vi "plcHMI_rev5.vi"() -> ()   [LabVIEW 2020]
doc: "ADS continuos synchronous write example using base blocks. \n\nThe client writes data synchronously and does wait for the respose from server."
uses:
  Agilent/AgilentTotalCluster.ctl
  Agilent/AgilentControl.ctl
  Agilent/Channel Config.ctl
  <vilib>/Platform/TimedLoop/XDataNode/timing_clust.ctl
  <vilib>/Platform/TimedLoop/XDataNode/nitl_modes.ctl
  <vilib>/Platform/TimedLoop/XDataNode/wakeup.ctl
  <userlib>/Beckhoff-LabVIEW-Interface/_DependsOn/With TypeResolving/Write Sync Single TypeResolved.vi
  <userlib>/Beckhoff-LabVIEW-Interface/_DependsOn/With TypeResolving/Read Sync Single TypeResolved.vi
  <vilib>/Platform/TimedLoop/XDataNode/XDataNode.xnode
  <vilib>/Platform/TimedLoop/XDataNode/XDNodeRunTimeDep.lvlib
panel:
  in  "Tab Control":T1(tab)
  out "error out":errorcluster
  in  "Symbol file path - MUST BE ENTERED\nLoad \"ADS Write AND Read Symbols REV X.X.xml\"":path
  out "bHasMached":bool
  out "Write Status":bool
  out "Read Status":bool
  in  "EXIT HMI":bool caption="STOP HMI\nEXIT HMI"
  out "Internal TwinCAT Handle ID Maps":dbl format="%#_12g"
  in  "802L TDK PSU Voltage Rating (abs(Volts))":i32=12000 min=1 max=50000
  in  "802L TDL PSU Peak Power (J/s)":i32=9000 min=1 max=50000
  in  "HVPS Model":u16(ring) items=["802L-12kV,9000J/s", "802L+50kV,9000J/s", "Other"]
  out "Test Interval Fault":bool
  in  "Cycle Time (Sec)":i32=15 min=0
  in  "Voltage Held by PSU":bool
  in  "Log Capacitor Voltage":bool
  in  "Log Temperature Data":bool
  out "Time Since Last Shot":string caption="Elapsed Time Text"
  in  "Duty Cycle":dbl
  in  "Current Control":bool
  out "Expected Voltage":i16
  in  "Dump":bool
  out "EOC":bool
  out "Maximum Test Number Reached":bool
  out "SCR Ready":bool
  in  "START":bool
  in  "STOP":bool
  in  "Hold":bool
  in  "Charge":bool
  in  "Shot":bool
  in  "HV Switch Mode":bool
  in  "CLEAR FAULT":bool
  in  "Manual/Auto":bool=TRUE
  out "Test Interval (Sec)":i32=15 min=0
  in  "Capacitance (uF)":sgl=1e-13 min=0 max=10000 format="%#_6f"
  in  "Target Charge Volt (V) - Min 1500V - TEMPORARY LIMIT 12kV":i32 min=-12000 max=12000 step=1
  out "Estimated Charge Time (seconds)":sgl
  in  "Hold Time Before Shot (seconds)":sgl max=1000
  in  "Max Number of Shots (Test intervals)":i16=1 min=1
  out "Shot Number":i16
  out "Charge Fault":bool=TRUE
  out "Discharge Fault":bool=TRUE
  out "Hold Fault":bool=TRUE
  out "Cap 1 Temp\nExceeded Fault":bool=TRUE
  out "Ambient Temp\nExceeded Fault":bool=TRUE
  out "PSU Fault":bool=TRUE
  out "Control Sys Fault":bool=TRUE
  out "test Running":bool
  out "Test State":string
  out "Cap 1 Voltage":i16
  out "Cap 1 Temperature":i16
  in  "Capacitor Voltage Data Log File Path (.xlsx)":path
  out "Load Temperature":i16
  out "Soft Dump Temp":i16
  out "Ambient Temp":i16
  out "Waveform Chart - Capacitor Voltage (Probe, abs(Volts))":dbl(graph)
  in  "Manual Charge Time (seconds)":sgl max=90
  in  "Reset Test Number":bool
  in  "Cap 1 Fault Temp (Cel)":i16 min=0 max=125
  in  "Capacitor Temperature Data Log File Path (.xlsx)":path
  out "Cap 1 Voltage (HVPS)":i16
  out "Capacitor Voltage":cluster{dbl, dbl}(graph)
  out "EOC":i16(graph)
  out "Soft Exception":bool
  out "PSU HV FB Fault":bool
  out "Charge FB Fault":bool
  out "Softdump FB Fault":bool
  out "SCR FB":i16(graph)
  out "Spark Gap Voltage":i16(graph)
  in  "CH4 Vertical Units":string(combo)="V"
  in  "CH4 Vertical Units/div":dbl=2.0
  in  "Toggle Scope Scale":bool
  in  "CH1 Vertical Units/div":dbl=2.0
  in  "CH1 Vertical Units":string(combo)="V"
  in  "Horizontal Units":enum16{"us", "ms", "s"}(ring)
  in  "Horizontal Units/div":dbl=200.0
  out "Download":bool
  in  "Single":bool
  in  "Stop":bool
  out "Scope Trig":bool
  in  "Agilent Array":T2[](array[typedef])
  out "Process Step":u8
  out "Stop Loops":bool
  # "CONFIGURATION"
  # "Press STOP HMI instead of\nLabView Abort Execution"
  # "PSU V Rating, Peak Power\nactive when OTHER\nis selected"
  # "INPUT VARIABLES - For TDK Lambda 802L\nMust be written to before START"
  # "FAULT STATUSES"
  # "Set to -1 for automated\nfull charge to setpoint"
  # "MANUAL CONTROLS"
  # "Does not record during \"wait\" and appends to data file. Must be named with .xlsx"
  # "HV Switch Configuration"
  # "Records during \"Test Running.\" Must be named with .xlsx"
  # "Control Sys Faults"
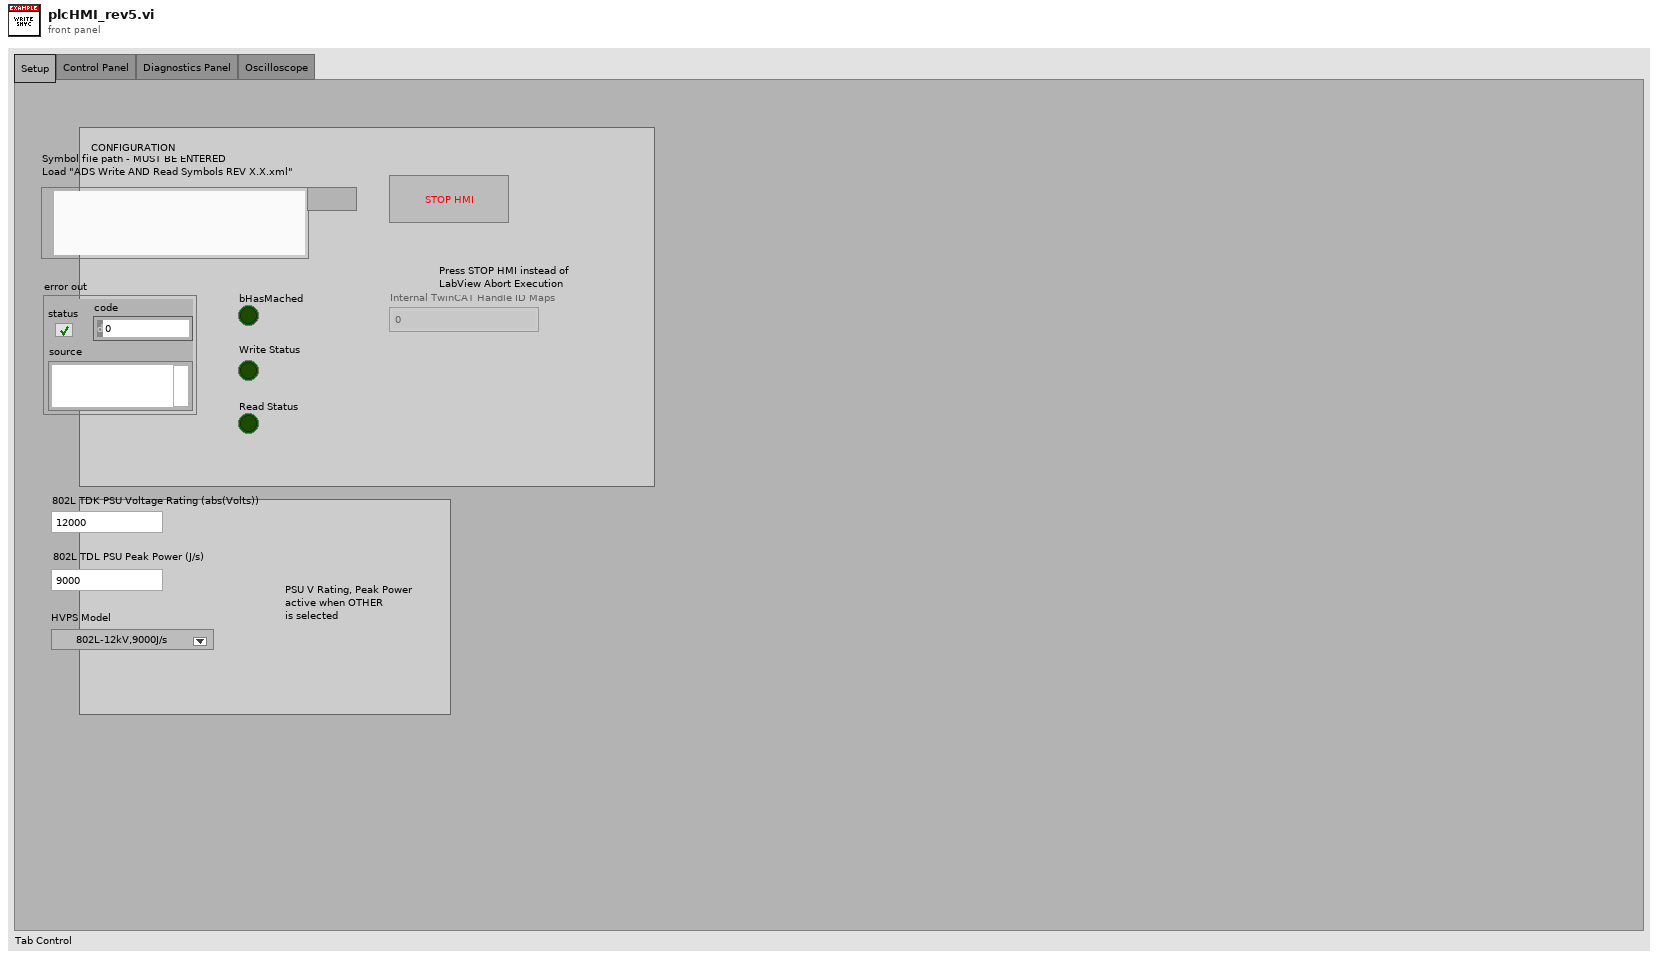
[diagram p1: front panel]
types:
  T1 = enum32{"Setup", "Control Panel", "Diagnostics Panel", "Oscilloscope"}
  T2 = typedef "AgilentTotalCluster.ctl" = cluster{"Agilent Graph":waveform(dbl)[], "Agilent Control":T3, "Agilent Setup Error":errorcluster, "Agilent Present":bool, "Enabled":bool}
  T3 = typedef "AgilentControl.ctl" = cluster{"Trig?":bool, "VISA session":refnum<visa-resource-name>, "Setup to Load":string, "Timeout (ms)":u32, "Desired Samp":enum32{"100", "250", "500", "1000", "2000", "5000", "10000", "20000", "50000", "100000", "200000", "500000", "1000000", "2000000", "4000000", "8000000"}, "Captured Samp":i32, "Desired Channels":T4[]}
  T4 = typedef "Channel Config.ctl" = cluster{"Chan Index":enum16{"Channel1", "Channel2", "Channel3", "Channel4", "MATH"}, "Name":string, "Samples":i32}
  T5 = typedef "XDNodeRunTimeDep.lvlib/timing_clust.ctl" = cluster{"Expected End [f-1]":u64, "Actual End [f-1]":u64, "Finished Late? [f-1]":bool, "Expected End [i-1]":u64, "Actual End [i-1]":u64, "Finished Late? [i-1]":bool, "Expected Start [i]":u64, "Actual Start [i]":u64, "Expected Start [f]":u64, "Actual Start [f]":u64, "Source Name":string, "Structure Name":string, "Period":i64, "Deadline":i64, "Offset":i64, "Start":i64, "Priority":i32, "Timeout":i32, "Mode":T6, "Wakeup Reason":T7, "Error":errorcluster, "Source Type":string, "Secondary Source Type":string, "Global End Time":u64, "Global Start Time":u64, "Frame Duration":u64, "Iteration Duration":u64, "Assigned CPU":i32, "I/O Scan Engine Mode":u32}
  T6 = typedef "XDNodeRunTimeDep.lvlib/nitl_modes.ctl" = enum32{"No Change", "Process missed periods, maintain original phase", "Discard missed periods, maintain original phase", "Process missed periods, ignore original phase", "Discard missed periods, ignore original phase"}
  T7 = typedef "XDNodeRunTimeDep.lvlib/wakeup.ctl" = enum32{"Normal", "Aborted", "Asynchronous wakeup", "Timing source error", "Timed loop error", "Timeout"}
  T8 = cluster{"Agilent Array[0]":T2, "Agilent Array[1]":T2, "Agilent Array[2]":T2, "Agilent Array[3]":T2, "Agilent Array[4]":T2, "Agilent Array[5]":T2, "Agilent Array[6]":T2, "Agilent Array[7]":T2, "Agilent Array[8]":T2}
  T9 = enum32{"100", "250", "500", "1000", "2000", "5000", "10000", "20000", "50000", "100000", "200000", "500000", "1000000", "2000000", "4000000", "8000000"}
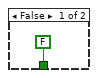
[diagram p2: hidden frame]
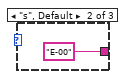
[diagram p5: hidden frame]
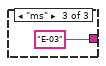
[diagram p6: hidden frame]
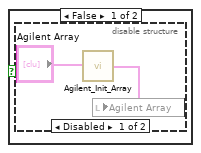
[diagram p7: hidden frame]
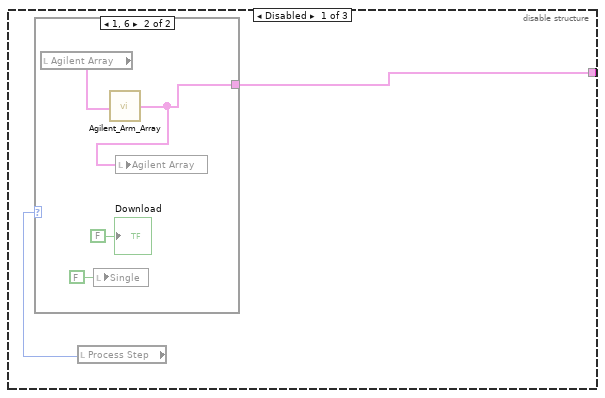
[diagram p11: hidden frame]
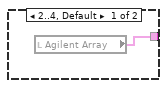
[diagram p12: hidden frame]
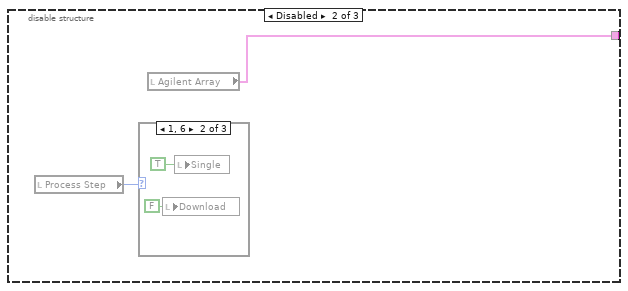
[diagram p13: hidden frame]
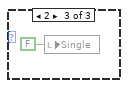
[diagram p15: hidden frame]
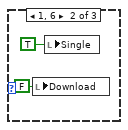
[diagram p17: hidden frame]
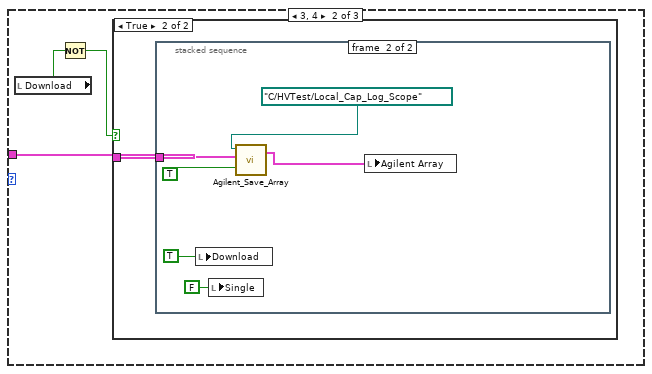
[diagram p19: hidden frame]
diagram:
  w91 = u16 17 items=["SyncLatest"=17, "AsyncLatest"=33] ("WriterMode")
  w161 = u16 33 items=["SyncLatest"=17, "AsyncLatest"=33] ("WriterMode")
  w201 = u16 33 items=["SyncLatest"=17, "AsyncLatest"=33] ("WriterMode")
  w220 = u16 33 items=["SyncLatest"=17, "AsyncLatest"=33] ("WriterMode")
  w239 = u16 33 items=["SyncLatest"=17, "AsyncLatest"=33] ("WriterMode")
  w258 = u16 33 items=["SyncLatest"=17, "AsyncLatest"=33] ("WriterMode")
  w277 = u16 33 items=["SyncLatest"=17, "AsyncLatest"=33] ("WriterMode")
  w296 = u16 17 items=["SyncLatest"=17, "AsyncLatest"=33] ("WriterMode")
  w315 = u16 17 items=["SyncLatest"=17, "AsyncLatest"=33] ("WriterMode")
  w334 = u16 17 items=["SyncLatest"=17, "AsyncLatest"=33] ("WriterMode")
  w353 = u16 17 items=["SyncLatest"=17, "AsyncLatest"=33] ("WriterMode")
  w372 = u16 17 items=["SyncLatest"=17, "AsyncLatest"=33] ("WriterMode")
  w391 = u16 17 items=["SyncLatest"=17, "AsyncLatest"=33] ("WriterMode")
  w410 = u16 17 items=["SyncLatest"=17, "AsyncLatest"=33] ("WriterMode")
  w425 = u16 17 items=["SyncLatest"=17, "AsyncLatest"=33] ("WriterMode")
  # "Variables/ Control"
  # "Documentation:\nCode separated vertically into two main sections - Write and read\nThey are further separated into BOOL and numeric\nThe OR gates wire all the error lines and the EXIT HMI button to a WHILE LOOP STOP\nThere current delay time on the routine is 100ms\nAll the AND gates connect the typecast resolve lines to the bHasMatched indicator\nThe second and third set of AND gates connect the write statuses to the Write Status indicator\nThe same is done for the read status indicator"
  # "WRITE NUMERICS"
  # "WRITE BOOLS"
  # "Select Symbol N"
  # "Read Initialization"
  # "Release \nTypeResolver"
  # "Release Writer"
  # "Send Request"
  # "Init \nTypeResolver"
  # "Init Writer"
  # "Select Symbol"
  # "Initialization"
  # "Call Release handle block\nat the end, when all nodes\nhave finished their execution"
  # "There must be only one release\nafter every init block.\nRelease block must be called\nalways at the end."
  # "Release"
  # "Symbol Interface"
  n1 = disable-structure shown="Enabled" {
    disable-tunnel: [w431 _] -> w429
    disable-tunnel: [w430 w433] -> w428
    frame Disabled {
      # "Using Symbol Interface"
      n2 = call <userlib>:"Symbol Interface.vi"() -> ("PortInfo"=w430:string, "error out"=w431:errorcluster)  [unwired: 14 in]
    }
    frame Enabled {
      # "Using Symbol File"
      n3 = Path To String(path="Symbol file path - MUST BE ENTERED\nLoad \"ADS Write AND Read Symbols REV X.X.xml\"") -> (string=w433:string)
    }
  }
  n4 = call <userlib>:"Init.vi"("XMLDescription"=w428, "error in (no error)"=w429) -> ("Handle"=w41:u32, "ReadGrpSymbols"=w5:string[], "WriteGrpSymbols"=w29:string[], "error out"=w7:errorcluster)  [unwired: 9 in, 1 out]
  n5 = Index Array(array=w29, index=0) -> (element=w18:string)
  n6 = Index Array(array=w29, index=21) -> (element=w28:string)
  n7 = Index Array(array=w29, index=20) -> (element=w34:string)
  n8 = Index Array(array=w29, index=14) -> (element=w8:string)
  n9 = Index Array(array=w29, index=9) -> (element=w278:string)
  n10 = Index Array(array=w29, index=10) -> (element=w259:string)
  n11 = Index Array(array=w29, index=12) -> (element=w221:string)
  n12 = Index Array(array=w29, index=11) -> (element=w240:string)
  n13 = Index Array(array=w29, index=13) -> (element=w202:string)
  n14 = Index Array(array=w29, index=18) -> (element=w42:string)
  n15 = Index Array(array=w29, index=19) -> (element=w35:string)
  n16 = Index Array(array=w29, index=7) -> (element=w297:string)
  n17 = Index Array(array=w29, index=2) -> (element=w392:string)
  n18 = Index Array(array=w29, index=3) -> (element=w373:string)
  n19 = Index Array(array=w29, index=5) -> (element=w335:string)
  n20 = Index Array(array=w29, index=4) -> (element=w354:string)
  n21 = Index Array(array=w29, index=6) -> (element=w316:string)
  n22 = Index Array(array=w29, index=1) -> (element=w411:string)
  n23 = Index Array(array=w29, index=16) -> (element=w11:string)
  n24 = Index Array(array=w29, index=8) -> (element=w90:string)
  n25 = Index Array(array=w29, index=15) -> (element=w162:string)
  n26 = Index Array(array=w29, index=17) -> (element=w13:string)
  n27 = call <userlib>:"Init Writer.vi"("Handle"=w41, "SymbolName"=w278, "WriterMode"=w277, "error constant"=w7) -> ("Handle"=w273:u32, "SymbolName"=w272:string, "WriterMode"=w271:u16, "WriteHandle"=w269:u32, "error IO"=w270:errorcluster)  [unwired: 7 in]
  n28 = call <userlib>:"Init Writer.vi"("Handle"=w41, "SymbolName"=w259, "WriterMode"=w258, "error constant"=w7) -> ("Handle"=w257:u32, "SymbolName"=w256:string, "WriterMode"=w255:u16, "WriteHandle"=w254:u32, "error IO"=w253:errorcluster)  [unwired: 7 in]
  n29 = call <userlib>:"Init Writer.vi"("Handle"=w41, "SymbolName"=w221, "WriterMode"=w220, "error constant"=w7) -> ("Handle"=w219:u32, "SymbolName"=w218:string, "WriterMode"=w217:u16, "WriteHandle"=w216:u32, "error IO"=w215:errorcluster)  [unwired: 7 in]
  n30 = call <userlib>:"Init Type.vi"("Handle"=w41, "SymbolName"=w278, "error in"=w7) -> ("Handle"=w262:u32, "TypeHdl"=w261:u32, "error IO"=w260:errorcluster)  [unwired: 7 in, 3 out]
  n31 = call <userlib>:"Init Type.vi"("Handle"=w41, "SymbolName"=w259, "error in"=w7) -> ("Handle"=w252:u32, "TypeHdl"=w251:u32, "error IO"=w250:errorcluster)  [unwired: 7 in, 3 out]
  n32 = call <userlib>:"Init Writer.vi"("Handle"=w41, "SymbolName"=w240, "WriterMode"=w239, "error constant"=w7) -> ("Handle"=w238:u32, "SymbolName"=w237:string, "WriterMode"=w236:u16, "WriteHandle"=w235:u32, "error IO"=w234:errorcluster)  [unwired: 7 in]
  n33 = call <userlib>:"Init Type.vi"("Handle"=w41, "SymbolName"=w221, "error in"=w7) -> ("Handle"=w214:u32, "TypeHdl"=w213:u32, "error IO"=w212:errorcluster)  [unwired: 7 in, 3 out]
  n34 = call <userlib>:"Init Writer.vi"("Handle"=w41, "SymbolName"=w202, "WriterMode"=w201, "error constant"=w7) -> ("Handle"=w200:u32, "SymbolName"=w199:string, "WriterMode"=w198:u16, "WriteHandle"=w197:u32, "error IO"=w196:errorcluster)  [unwired: 7 in]
  n35 = call <userlib>:"Init Type.vi"("Handle"=w41, "SymbolName"=w240, "error in"=w7) -> ("Handle"=w233:u32, "TypeHdl"=w232:u32, "error IO"=w231:errorcluster)  [unwired: 7 in, 3 out]
  n36 = call <userlib>:"Init Type.vi"("Handle"=w41, "SymbolName"=w202, "error in"=w7) -> ("Handle"=w195:u32, "TypeHdl"=w194:u32, "error IO"=w193:errorcluster)  [unwired: 7 in, 3 out]
  n37 = call <userlib>:"Init Writer.vi"("Handle"=w41, "SymbolName"=w297, "WriterMode"=w296, "error constant"=w7) -> ("Handle"=w295:u32, "SymbolName"=w294:string, "WriterMode"=w293:u16, "WriteHandle"=w292:u32, "error IO"=w291:errorcluster)  [unwired: 7 in]
  n38 = call <userlib>:"Init Writer.vi"("Handle"=w41, "SymbolName"=w392, "WriterMode"=w391, "error constant"=w7) -> ("Handle"=w387:u32, "SymbolName"=w386:string, "WriterMode"=w385:u16, "WriteHandle"=w383:u32, "error IO"=w384:errorcluster)  [unwired: 7 in]
  n39 = call <userlib>:"Init Writer.vi"("Handle"=w41, "SymbolName"=w373, "WriterMode"=w372, "error constant"=w7) -> ("Handle"=w371:u32, "SymbolName"=w370:string, "WriterMode"=w369:u16, "WriteHandle"=w368:u32, "error IO"=w367:errorcluster)  [unwired: 7 in]
  n40 = call <userlib>:"Init Writer.vi"("Handle"=w41, "SymbolName"=w335, "WriterMode"=w334, "error constant"=w7) -> ("Handle"=w333:u32, "SymbolName"=w332:string, "WriterMode"=w331:u16, "WriteHandle"=w330:u32, "error IO"=w329:errorcluster)  [unwired: 7 in]
  n41 = call <userlib>:"Init Type.vi"("Handle"=w41, "SymbolName"=w297, "error in"=w7) -> ("Handle"=w290:u32, "TypeHdl"=w289:u32, "error IO"=w288:errorcluster)  [unwired: 7 in, 3 out]
  n42 = call <userlib>:"Init Type.vi"("Handle"=w41, "SymbolName"=w392, "error in"=w7) -> ("Handle"=w376:u32, "TypeHdl"=w375:u32, "error IO"=w374:errorcluster)  [unwired: 7 in, 3 out]
  n43 = call <userlib>:"Init Type.vi"("Handle"=w41, "SymbolName"=w373, "error in"=w7) -> ("Handle"=w366:u32, "TypeHdl"=w365:u32, "error IO"=w364:errorcluster)  [unwired: 7 in, 3 out]
  n44 = call <userlib>:"Init Writer.vi"("Handle"=w41, "SymbolName"=w354, "WriterMode"=w353, "error constant"=w7) -> ("Handle"=w352:u32, "SymbolName"=w351:string, "WriterMode"=w350:u16, "WriteHandle"=w349:u32, "error IO"=w348:errorcluster)  [unwired: 7 in]
  n45 = call <userlib>:"Init Type.vi"("Handle"=w41, "SymbolName"=w335, "error in"=w7) -> ("Handle"=w328:u32, "TypeHdl"=w327:u32, "error IO"=w326:errorcluster)  [unwired: 7 in, 3 out]
  n46 = call <userlib>:"Init Writer.vi"("Handle"=w41, "SymbolName"=w316, "WriterMode"=w315, "error constant"=w7) -> ("Handle"=w314:u32, "SymbolName"=w313:string, "WriterMode"=w312:u16, "WriteHandle"=w311:u32, "error IO"=w310:errorcluster)  [unwired: 7 in]
  n47 = call <userlib>:"Init Type.vi"("Handle"=w41, "SymbolName"=w354, "error in"=w7) -> ("Handle"=w347:u32, "TypeHdl"=w346:u32, "error IO"=w345:errorcluster)  [unwired: 7 in, 3 out]
  n48 = call <userlib>:"Init Type.vi"("Handle"=w41, "SymbolName"=w316, "error in"=w7) -> ("Handle"=w309:u32, "TypeHdl"=w308:u32, "error IO"=w307:errorcluster)  [unwired: 7 in, 3 out]
  n49 = call <userlib>:"Init Writer.vi"("Handle"=w41, "SymbolName"=w411, "WriterMode"=w410, "error constant"=w7) -> ("Handle"=w409:u32, "SymbolName"=w408:string, "WriterMode"=w407:u16, "WriteHandle"=w406:u32, "error IO"=w405:errorcluster)  [unwired: 7 in]
  n50 = call <userlib>:"Init Type.vi"("Handle"=w41, "SymbolName"=w411, "error in"=w7) -> ("Handle"=w404:u32, "TypeHdl"=w403:u32, "error IO"=w402:errorcluster)  [unwired: 7 in, 3 out]
  n51 = call <userlib>:"Init Writer.vi"("Handle"=w41, "SymbolName"=w18, "WriterMode"=w425, "error constant"=w7) -> ("Handle"=w424:u32, "SymbolName"=w423:string, "WriterMode"=w422:u16, "WriteHandle"=w421:u32, "error IO"=w420:errorcluster)  [unwired: 7 in]
  n52 = call <userlib>:"Init Type.vi"("Handle"=w41, "SymbolName"=w18, "error in"=w7) -> ("Handle"=w419:u32, "TypeHdl"=w418:u32, "error IO"=w413:errorcluster)  [unwired: 7 in, 3 out]
  n53 = call <userlib>:"Init Writer.vi"("Handle"=w41, "SymbolName"=w162, "WriterMode"=w161, "error constant"=w7) -> ("Handle"=w157:u32, "SymbolName"=w156:string, "WriterMode"=w155:u16, "WriteHandle"=w147:u32, "error IO"=w154:errorcluster)  [unwired: 7 in]
  n54 = call <userlib>:"Init Type.vi"("Handle"=w41, "SymbolName"=w162, "error in"=w7) -> ("Handle"=w152:u32, "TypeHdl"=w150:u32, "error IO"=w151:errorcluster)  [unwired: 7 in, 3 out]
  n55 = Index Array(array=w5, index=2) -> (element=w143:string)
  n56 = Index Array(array=w5, index=4) -> (element=w139:string)
  n57 = call <userlib>:"Init Writer.vi"("Handle"=w41, "SymbolName"=w90, "WriterMode"=w91, "error constant"=w7) -> ("Handle"=w89:u32, "SymbolName"=w88:string, "WriterMode"=w87:u16, "WriteHandle"=w86:u32, "error IO"=w85:errorcluster)  [unwired: 7 in]
  n58 = Index Array(array=w5, index=1) -> (element=w179:string)
  n59 = Index Array(array=w5, index=21) -> (element=w56:string)
  n60 = Index Array(array=w5, index=22) -> (element=w53:string)
  n61 = call <userlib>:"Init Type.vi"("Handle"=w41, "SymbolName"=w90, "error in"=w7) -> ("Handle"=w84:u32, "TypeHdl"=w83:u32, "error IO"=w82:errorcluster)  [unwired: 7 in, 3 out]
  n62 = Index Array(array=w5, index=0) -> (element=w178:string)
  n63 = Index Array(array=w5, index=3) -> (element=w140:string)
  n64 = Index Array(array=w5, index=20) -> (element=w61:string)
  n65 = Index Array(array=w5, index=23) -> (element=w52:string)
  n66 = Index Array(array=w5, index=16) -> (element=w145:string)
  n67 = Index Array(array=w5, index=24) -> (element=w50:string)
  n68 = Index Array(array=w5, index=28) -> (element=w3:string)
  n69 = Index Array(array=w5, index=11) -> (element=w167:string)
  n70 = Index Array(array=w5, index=10) -> (element=w168:string)
  n71 = Index Array(array=w5, index=17) -> (element=w64:string)
  n72 = Index Array(array=w5, index=18) -> (element=w63:string)
  n73 = Index Array(array=w5, index=13) -> (element=w165:string)
  n74 = Index Array(array=w5, index=27) -> (element=w22:string)
  n75 = Index Array(array=w5, index=12) -> (element=w166:string)
  n76 = Index Array(array=w5, index=15) -> (element=w163:string)
  n77 = Index Array(array=w5, index=19) -> (element=w62:string)
  n78 = Index Array(array=w5, index=26) -> (element=w23:string)
  n79 = Index Array(array=w5, index=5) -> (element=w75:string)
  n80 = Index Array(array=w5, index=6) -> (element=w133:string)
  n81 = Index Array(array=w5, index=9) -> (element=w177:string)
  n82 = Index Array(array=w5, index=14) -> (element=w164:string)
  n83 = Index Array(array=w5, index=8) -> (element=w135:string)
  n84 = Index Array(array=w5, index=25) -> (element=w39:string)
  n85 = Index Array(array=w5, index=7) -> (element=w134:string)
  n86 = node-c288(i64 10 ("Period")) -> (w99:T5)  [unwired: 2 in]
  n87 = timed-loop {
    tunnel: w424 -> [w741]
    tunnel: w423 -> [w740]
    tunnel: w422 -> [w739]
    tunnel: w421 -> [w738]
    tunnel: w419 -> [w983]
    tunnel: w418 -> [w982]
    tunnel: [w736] -> w417
    tunnel: [w735] -> w416
    tunnel: [w981] -> w415
    tunnel: [w980] -> w414
    tunnel: w409 -> [w978]
    tunnel: w408 -> [w977]
    tunnel: w407 -> [w976]
    tunnel: w406 -> [w975]
    tunnel: w404 -> [w973]
    tunnel: w403 -> [w972]
    tunnel: [w970] -> w400
    tunnel: [w969] -> w399
    tunnel: [w968] -> w397
    tunnel: [w967] -> w396
    tunnel: w387 -> [w966]
    tunnel: w386 -> [w965]
    tunnel: w385 -> [w964]
    tunnel: w383 -> [w962]
    tunnel: [w961] -> w382
    tunnel: [w960] -> w381
    tunnel: [w959] -> w378
    tunnel: [w958] -> w377
    tunnel: w376 -> [w957]
    tunnel: w375 -> [w956]
    tunnel: w371 -> [w954]
    tunnel: w370 -> [w953]
    tunnel: w369 -> [w952]
    tunnel: w368 -> [w951]
    tunnel: w366 -> [w949]
    tunnel: w365 -> [w948]
    tunnel: [w946] -> w362
    tunnel: [w945] -> w361
    tunnel: [w944] -> w359
    tunnel: [w943] -> w358
    tunnel: w352 -> [w942]
    tunnel: w351 -> [w941]
    tunnel: w350 -> [w940]
    tunnel: w349 -> [w939]
    tunnel: w347 -> [w937]
    tunnel: w346 -> [w936]
    tunnel: [w934] -> w343
    tunnel: [w933] -> w342
    tunnel: [w932] -> w340
    tunnel: [w931] -> w339
    tunnel: w333 -> [w930]
    tunnel: w332 -> [w929]
    tunnel: w331 -> [w928]
    tunnel: w330 -> [w927]
    tunnel: w328 -> [w925]
    tunnel: w327 -> [w924]
    tunnel: [w922] -> w324
    tunnel: [w921] -> w323
    tunnel: [w920] -> w321
    tunnel: [w919] -> w320
    tunnel: w314 -> [w918]
    tunnel: w313 -> [w917]
    tunnel: w312 -> [w916]
    tunnel: w311 -> [w915]
    tunnel: w309 -> [w913]
    tunnel: w308 -> [w912]
    tunnel: [w910] -> w305
    tunnel: [w909] -> w304
    tunnel: [w908] -> w302
    tunnel: [w907] -> w301
    tunnel: w295 -> [w906]
    tunnel: w294 -> [w905]
    tunnel: w293 -> [w904]
    tunnel: w292 -> [w903]
    tunnel: w290 -> [w901]
    tunnel: w289 -> [w900]
    tunnel: [w898] -> w286
    tunnel: [w897] -> w285
    tunnel: [w896] -> w283
    tunnel: [w895] -> w282
    tunnel: w273 -> [w894]
    tunnel: w272 -> [w893]
    tunnel: w271 -> [w892]
    tunnel: w269 -> [w890]
    tunnel: [w889] -> w268
    tunnel: [w888] -> w267
    tunnel: [w887] -> w264
    tunnel: [w886] -> w263
    tunnel: w262 -> [w885]
    tunnel: w261 -> [w884]
    tunnel: w257 -> [w882]
    tunnel: w256 -> [w881]
    tunnel: w255 -> [w880]
    tunnel: w254 -> [w879]
    tunnel: w252 -> [w877]
    tunnel: w251 -> [w876]
    tunnel: [w874] -> w248
    tunnel: [w873] -> w247
    tunnel: [w872] -> w245
    tunnel: [w871] -> w244
    tunnel: w238 -> [w870]
    tunnel: w237 -> [w869]
    tunnel: w236 -> [w868]
    tunnel: w235 -> [w867]
    tunnel: w233 -> [w865]
    tunnel: w232 -> [w864]
    tunnel: [w862] -> w229
    tunnel: [w861] -> w228
    tunnel: [w860] -> w226
    tunnel: [w859] -> w225
    tunnel: w219 -> [w858]
    tunnel: w218 -> [w857]
    tunnel: w217 -> [w856]
    tunnel: w216 -> [w855]
    tunnel: w214 -> [w853]
    tunnel: w213 -> [w852]
    tunnel: [w850] -> w210
    tunnel: [w849] -> w209
    tunnel: [w848] -> w207
    tunnel: [w847] -> w206
    tunnel: w200 -> [w846]
    tunnel: w199 -> [w845]
    tunnel: w198 -> [w844]
    tunnel: w197 -> [w843]
    tunnel: w195 -> [w841]
    tunnel: w194 -> [w840]
    tunnel: [w838] -> w191
    tunnel: [w837] -> w190
    tunnel: [w836] -> w188
    tunnel: [w835] -> w187
    tunnel: w179 -> [w834]
    tunnel: w178 -> [w833]
    tunnel: w177 -> [w832]
    tunnel: [w831] -> w128
    tunnel: w168 -> [w830]
    tunnel: w167 -> [w829]
    tunnel: w166 -> [w828]
    tunnel: w165 -> [w827]
    tunnel: w164 -> [w826]
    tunnel: w163 -> [w825]
    tunnel: [w824] -> w96
    tunnel: [w823] -> w127
    tunnel: [w822] -> w126
    tunnel: [w821] -> w125
    tunnel: [w820] -> w124
    tunnel: [w764] -> w123
    tunnel: [w762] -> w122
    shift-right: [w665] -> w427
    shift-left: w420 -> [w737]
    shift-right: [w664] -> w426
    shift-left: w413 -> [w979]
    shift-right: [w662] -> w398
    shift-left: w405 -> [w974]
    shift-right: [w661] -> w395
    shift-left: w402 -> [w971]
    shift-right: [w659] -> w380
    shift-left: w384 -> [w963]
    shift-right: [w658] -> w379
    shift-left: w374 -> [w955]
    shift-right: [w656] -> w360
    shift-left: w367 -> [w950]
    shift-right: [w655] -> w357
    shift-left: w364 -> [w947]
    shift-right: [w653] -> w341
    shift-left: w348 -> [w938]
    shift-right: [w652] -> w338
    shift-left: w345 -> [w935]
    shift-right: [w650] -> w322
    shift-left: w329 -> [w926]
    shift-right: [w649] -> w319
    shift-left: w326 -> [w923]
    shift-right: [w647] -> w303
    shift-left: w310 -> [w914]
    shift-right: [w646] -> w300
    shift-left: w307 -> [w911]
    shift-right: [w644] -> w284
    shift-left: w291 -> [w902]
    shift-right: [w643] -> w281
    shift-left: w288 -> [w899]
    shift-right: [w642] -> w266
    shift-left: w270 -> [w891]
    shift-right: [w641] -> w265
    shift-left: w260 -> [w883]
    shift-right: [w639] -> w246
    shift-left: w253 -> [w878]
    shift-right: [w638] -> w243
    shift-left: w250 -> [w875]
    shift-right: [w636] -> w227
    shift-left: w234 -> [w866]
    shift-right: [w635] -> w224
    shift-left: w231 -> [w863]
    shift-right: [w633] -> w208
    shift-left: w215 -> [w854]
    shift-right: [w632] -> w205
    shift-left: w212 -> [w851]
    shift-right: [w630] -> w189
    shift-left: w196 -> [w842]
    shift-right: [w629] -> w186
    shift-left: w193 -> [w839]
    tunnel: w157 -> [w804]
    tunnel: w156 -> [w803]
    tunnel: w155 -> [w802]
    tunnel: [w800] -> w17
    tunnel: [w799] -> w153
    tunnel: w152 -> [w798]
    tunnel: w150 -> [w796]
    tunnel: [w795] -> w149
    tunnel: [w794] -> w148
    tunnel: w147 -> [w793]
    tunnel: w145 -> [w792]
    tunnel: [w763] -> w121
    tunnel: [w786] -> w130
    tunnel: w7 -> [w785]
    tunnel: [w783] -> w129
    tunnel: w143 -> [w782]
    tunnel: w140 -> [w778]
    tunnel: w139 -> [w777]
    tunnel: [w768] -> w131
    tunnel: [w767] -> w132
    tunnel: w135 -> [w761]
    tunnel: w134 -> [w760]
    tunnel: w133 -> [w759]
    tunnel: [w746] -> w72
    tunnel: [w745] -> w71
    tunnel: [w744] -> w70
    timing: w99 -> [_]
    timing-out: [_] -> w98
    tunnel: w41 -> [w734]
    tunnel: [w627] -> w74
    tunnel: w89 -> [w622]
    tunnel: w88 -> [w621]
    tunnel: w87 -> [w620]
    tunnel: w86 -> [w619]
    tunnel: w84 -> [w617]
    tunnel: w83 -> [w616]
    tunnel: [w613] -> w81
    tunnel: [w612] -> w80
    tunnel: [w611] -> w79
    tunnel: [w610] -> w78
    tunnel: [w603] -> w73
    tunnel: w75 -> [w599]
    tunnel: [w598] -> w69
    tunnel: w64 -> [w594]
    tunnel: w63 -> [w589]
    tunnel: w62 -> [w588]
    tunnel: w61 -> [w587]
    tunnel: [w584] -> w60
    tunnel: [w582] -> w59
    tunnel: [w577] -> w58
    tunnel: [w576] -> w45
    tunnel: w56 -> [w574]
    tunnel: w53 -> [w549]
    tunnel: w52 -> [w548]
    tunnel: w50 -> [w541]
    tunnel: [w537] -> w49
    tunnel: [w536] -> w48
    tunnel: [w535] -> w47
    tunnel: [w534] -> w46
    tunnel: w42 -> [w533]
    tunnel: w41 -> [w446]
    tunnel: w7 -> [w532]
    tunnel: [w529] -> w33
    tunnel: [w528] -> _
    tunnel: w39 -> [w524]
    tunnel: [w520] -> w38
    tunnel: w35 -> [w519]
    tunnel: w34 -> [w518]
    tunnel: w7 -> [w495]
    tunnel: [w513] -> w32
    tunnel: [w512] -> w31
    tunnel: w28 -> [w499]
    tunnel: [w494] -> w27
    tunnel: w23 -> [w481]
    tunnel: w22 -> [w480]
    tunnel: [w475] -> w21
    tunnel: [w474] -> w2
    shift-right: [w472] -> w20
    shift-left: w154 -> [w801]
    shift-right: [w471] -> w19
    shift-left: w151 -> [w797]
    tunnel: w7 -> [w464]
    tunnel: [w461] -> w12
    shift-right: [w469] -> w15
    shift-left: w85 -> [w618]
    shift-right: [w468] -> w14
    shift-left: w82 -> [w615]
    tunnel: w13 -> [w463]
    tunnel: w11 -> [w456]
    tunnel: w7 -> [w455]
    tunnel: [w454] -> w10
    tunnel: w8 -> [w447]
    tunnel: w7 -> [w445]
    tunnel: [w444] -> w6
    tunnel: w3 -> [w438]
    tunnel: [w434] -> w1
    stop <- w439 stop-if-true
    # "Stop Loop on Error (OR gates)"
    # "Error Stop Loop AND"
    # "Typecast Match AND"
    # "Write Status AND"
    # "READ BOOLS"
    # "READ NUMERICS"
    # "STOP HMI via error or EXIT button"
    # "Check Read status and\nthen convert Variant \nto LabVIEW type (AND gates)"
    # "Sync Read Single"
    n88 = node-c288() -> (w628:errorcluster)  [unwired: 1 in]
    n89 = disable-structure shown="Enabled" {
      frame Enabled {
        n90 = flat-sequence {
          tunnel: [w1119] -> w1063
          tunnel: w1063 -> [w1138]
          frame #0 {
            n91 = disable-structure shown="Enabled" {
              frame Enabled {
                n92 = feedback #1(TRUE) -> (w1065:bool)
                n93 = And(x=TRUE, y=w1065) -> (x .and. y?=w1068:bool)
                n94 = case shown="True" w1068 {
                  tunnel: [FALSE FALSE] -> w1066
                  frame False {
                  }
                  frame True {
                    n95 = local read "Agilent Array"() -> (w1071:T2[])
                    n96 = call "Agilent_Init_Array.vi"("Agilent Array In"=w1071) -> ("Agilent Array Out"=w1072:T2[])
                    n97 = call "Agilent_Arm_Array.vi"("Agilent Array In"=w1072) -> ("Agilent Array Out"=w1070:T2[])
                    n98 = local write "Agilent Array"(w1070) -> ()
                  }
                }
                n99 = feedback-in #1(w1066) -> ()
              }
              frame Disabled {
              }
            }
          }
          frame #1 {
            n100 = case shown="True" "Toggle Scope Scale" {
              frame False {
              }
              frame True {
                n101 = Number To Decimal String(number="CH4 Vertical Units/div") -> (decimal integer string=w1078:string)  [unwired: 1 in]
                n102 = Number To Decimal String(number="Horizontal Units/div") -> (decimal integer string=w1086:string)  [unwired: 1 in]
                n103 = Number To Decimal String(number="CH1 Vertical Units/div") -> (decimal integer string=w1084:string)  [unwired: 1 in]
                n104 = case shown="\"us\"" "Horizontal Units" {
                  tunnel: ["E-06" "E-00" "E-03"] -> w1095
                  frame "us" {
                  }
                  frame "s", Default {
                  }
                  frame "ms" {
                  }
                }
                n105 = Concatenate Strings(":CHAN4:SCAL " ("write buffer"), w1078, "CH4 Vertical Units") -> (w1077:string)
                n106 = Concatenate Strings(":CHAN1:SCAL " ("write buffer"), w1084, "CH1 Vertical Units") -> (w1091:string)
                n107 = Concatenate Strings(":TIM:SCAL " ("write buffer"), w1086, w1095) -> (w1094:string)
                n108 = VISA Open(VISA resource name=refnum<visa-resource-name> "HV_Test_Scope") -> (VISA resource name=w1089:refnum<visa-resource-name>, error out=w1090:errorcluster)  [unwired: 4 in]
                n109 = VISA Write(VISA resource name=w1089, write buffer=w1094, error in (no error)=w1090) -> (VISA resource name out=w1098:refnum<visa-resource-name>, error out=w1097:errorcluster)  [unwired: 1 out]
                n110 = VISA Write(VISA resource name=w1098, write buffer=w1091, error in (no error)=w1097) -> (VISA resource name out=w1083:refnum<visa-resource-name>, error out=w1081:errorcluster)  [unwired: 1 out]
                n111 = VISA Write(VISA resource name=w1083, write buffer=w1077, error in (no error)=w1081) -> (VISA resource name out=w1082:refnum<visa-resource-name>, error out=w1080:errorcluster)  [unwired: 1 out]
                n112 = VISA Close(VISA resource name=w1082, error in (no error)=w1080) -> ()  [unwired: 1 out]
              }
            }
          }
          frame #2 {
            n113 = disable-structure shown="Enabled" {
              frame Enabled {
                n114 = case shown="True" "Stop" {
                  frame False {
                    n115 = disable-structure shown="Disabled" {
                      frame Disabled {
                        n116 = call "Agilent_Init_Array.vi"("Agilent Array In"="Agilent Array") -> ("Agilent Array Out"=w1105:T2[])
                        n117 = local write "Agilent Array"(w1105) -> ()
                      }
                      frame Enabled {
                      }
                    }
                  }
                  frame True {
                    n118 = VISA Open(VISA resource name=refnum<visa-resource-name> "HV_Test_Scope") -> (VISA resource name=w1111:refnum<visa-resource-name>, error out=w1112:errorcluster)  [unwired: 4 in]
                    n119 = VISA Write(VISA resource name=w1111, write buffer=":STOP", error in (no error)=w1112) -> (VISA resource name out=w1109:refnum<visa-resource-name>, error out=w1110:errorcluster)  [unwired: 1 out]
                    n120 = VISA Close(VISA resource name=w1109, error in (no error)=w1110) -> ()  [unwired: 1 out]
                  }
                }
              }
              frame Disabled {
              }
            }
            n121 = case shown="True" "Single" {
              frame False {
              }
              frame True {
                n122 = VISA Open(VISA resource name=refnum<visa-resource-name> "HV_Test_Scope") -> (VISA resource name=w1117:refnum<visa-resource-name>, error out=w1118:errorcluster)  [unwired: 4 in]
                n123 = VISA Write(VISA resource name=w1117, write buffer=":SINGLE", error in (no error)=w1118) -> (VISA resource name out=w1115:refnum<visa-resource-name>, error out=w1116:errorcluster)  [unwired: 1 out]
                n124 = VISA Close(VISA resource name=w1115, error in (no error)=w1116) -> ()  [unwired: 1 out]
              }
            }
          }
          frame #3 {
            n125 = disable-structure shown="Enabled" {
              disable-tunnel: [w1121 w1128 w1133] -> w1119
              frame Disabled {
                n126 = local read "Process Step"() -> (w1120:u8)
                n127 = case shown="1, 6" w1120 {
                  tunnel: [w1122 w1126] -> w1121
                  frame 2..4, Default {
                    n128 = local read "Agilent Array"() -> (w1122:T2[])
                  }
                  frame 1, 6 {
                    n129 = local read "Agilent Array"() -> (w1123:T2[])
                    n130 = local write "Single"(FALSE ("Single")) -> ()
                    n131 = call "Agilent_Arm_Array.vi"("Agilent Array In"=w1123) -> ("Agilent Array Out"=w1126:T2[])
                    n132 = local write "Agilent Array"(w1126) -> ()
                    "Download" <- FALSE ("Downloading")
                  }
                }
              }
              frame Disabled {
                n133 = local read "Process Step"() -> (w1127:u8)
                n134 = case shown="1, 6" w1127 {
                  frame 0, Default {
                  }
                  frame 1, 6 {
                    n135 = local write "Download"(FALSE ("Download")) -> ()
                    n136 = local write "Single"(TRUE ("Single")) -> ()
                  }
                  frame 2 {
                    n137 = local write "Single"(FALSE ("Single")) -> ()
                  }
                }
                n138 = local read "Agilent Array"() -> (w1128:T2[])
              }
              frame Enabled {
                n139 = local read "Process Step"() -> (w1132:u8)
                n140 = case shown="2, 7" w1132 {
                  frame 0, Default {
                  }
                  frame 1, 6 {
                    n141 = local write "Download"(FALSE ("Download")) -> ()
                    n142 = local write "Single"(TRUE ("Single")) -> ()
                  }
                  frame 2, 7 {
                    n143 = local write "Single"(FALSE ("Single")) -> ()
                  }
                }
                n144 = local read "Agilent Array"() -> (w1133:T2[])
              }
            }
          }
          frame #4 {
            n145 = local read "Process Step"() -> (w1137:u8)
            n146 = case shown="0" w1137 {
              tunnel: w1138 -> [_ w1141 w1154]
              frame Default {
              }
              frame 3, 4 {
                n147 = local read "Download"() -> (w1140:bool)
                n148 = Not(x=w1140) -> (.not. x?=w1139:bool)
                n149 = case shown="True" w1139 {
                  tunnel: w1141 -> [_ w1142]
                  frame False {
                  }
                  frame True {
                    n150 = stacked-sequence {
                      tunnel: w1142 -> [_ w1152]
                      frame #0 {
                        n151 = local read "Agilent Array"() -> (w1146:T2[])
                        n152 = Array To Cluster(array=w1146) -> (cluster=w1145:T8)
                        n153 = Unbundle By Name(w1145) -> ("Agilent Array[0].Agilent Control.Desired Samp"=w1143:T9)
                        n154 = call "GF_SetRecordLengthProperly.vi"("Num Samples"=w1143, "VISA resource name"=refnum<visa-resource-name> "HV_Test_Scope") -> ()  [unwired: 1 in, 2 out]
                      }
                      frame #1 {
                        n155 = local write "Download"(TRUE ("Downloading")) -> ()
                        n156 = local write "Single"(FALSE ("Single")) -> ()
                        n157 = call "Agilent_Save_Array.vi"("Agilent Download"=TRUE, "Agilent Array In"=w1152, "File Path"=path "C:/HVTest/Local_Cap_Log_Scope") -> ("Agilent Array Out"=w1150:T2[])  [unwired: 1 in, 1 out]
                        n158 = local write "Agilent Array"(w1150) -> ()
                      }
                    }
                  }
                }
              }
              frame 0 {
                n159 = local read "Maximum Test Number Reached"() -> (w1153:bool)
                n160 = case shown="True" w1153 {
                  tunnel: w1154 -> [_ w1157]
                  frame False {
                  }
                  frame True {
                    n161 = local read "Download"() -> (w1156:bool)
                    n162 = Not(x=w1156) -> (.not. x?=w1155:bool)
                    n163 = case shown="True" w1155 {
                      tunnel: w1157 -> [_ w1158]
                      frame False {
                      }
                      frame True {
                        n164 = stacked-sequence {
                          tunnel: w1158 -> [_ w1168]
                          frame #0 {
                            n165 = local read "Agilent Array"() -> (w1162:T2[])
                            n166 = Array To Cluster(array=w1162) -> (cluster=w1161:T8)
                            n167 = Unbundle By Name(w1161) -> ("Agilent Array[0].Agilent Control.Desired Samp"=w1159:T9)
                            n168 = call "GF_SetRecordLengthProperly.vi"("Num Samples"=w1159, "VISA resource name"=refnum<visa-resource-name> "HV_Test_Scope") -> ()  [unwired: 1 in, 2 out]
                          }
                          frame #1 {
                            n169 = local write "Download"(TRUE ("Downloading")) -> ()
                            n170 = local write "Single"(FALSE ("Single")) -> ()
                            n171 = call "Agilent_Save_Array.vi"("Agilent Download"=TRUE, "Agilent Array In"=w1168, "File Path"=path "C:/HVTest/Local_Cap_Log_Scope") -> ("Agilent Array Out"=w1166:T2[])  [unwired: 1 in, 1 out]
                            n172 = local write "Agilent Array"(w1166) -> ()
                          }
                        }
                      }
                    }
                  }
                }
              }
            }
          }
        }
      }
      frame Disabled {
      }
    }
    n173 = To Word Integer(number="Max Number of Shots (Test intervals)") -> (16bit integer=w450:i16)
    n174 = To Variant(anything=w450) -> (Variant=w449:variant)
    n175 = case shown="0, Default" "HVPS Model" {
      tunnel: ["802L TDK PSU Voltage Rating (abs(Volts))" 12000 50000] -> w742
      tunnel: ["802L TDL PSU Peak Power (J/s)" 9000 9000] -> w765
      frame 2 {
      }
      frame 0, Default {
      }
      frame 1 {
      }
    }
    n176 = call-poly <userlib>:"Write TypeResolved.vi"("Handle"=w446, "SymbolName"=w447, "WData"=w449, "error constant"=w445) -> ("Write Status?"=w441:bool, "Has Matched?"=w442:bool, "error out"=w444:errorcluster)  [unwired: 8 in, 1 out]
    n177 = To Single Precision Float(number="Manual Charge Time (seconds)") -> (single precision float=w458:sgl)
    n178 = To Variant(anything=w458) -> (Variant=w457:variant)
    n179 = flat-sequence {
      tunnel: w798 -> [w1266]
      tunnel: w796 -> [w1267]
      tunnel: w797 -> [w1268]
      tunnel: [w1268] -> w808
      tunnel: [w1267] -> w807
      tunnel: [w1266] -> w806
      tunnel: [w1265] -> w805
      tunnel: w765 -> [w1264]
      tunnel: [w1271] -> w471
      tunnel: [w1274] -> w794
      tunnel: [w1273] -> w795
      tunnel: [w1272] -> w473
      tunnel: w808 -> [w1277]
      tunnel: w807 -> [w1276]
      tunnel: w806 -> [w1275]
      tunnel: w805 -> [w1270]
      tunnel: [w1269] -> w691
      frame #0 {
        # "Write Data"
        n180 = To Long Integer(number=w1264) -> (32bit integer=w1263:i32)
        n181 = To Variant(anything=w1263) -> (Variant=w1265:variant)
      }
      frame #1 {
        # "Resolve To TC"
        n182 = call <userlib>:"Resolve To TC Type.vi"("Handle"=w1275, "TypHdl"=w1276, "WData"=w1270, "error in"=w1277) -> ("Handle"=w1273:u32, "TypHdl"=w1274:u32, "bHasMatched"=w1269:bool, "ADSWData"=w1272:variant, "error out"=w1271:errorcluster)  [unwired: 7 in]
      }
    }
    n183 = flat-sequence {
      tunnel: w877 -> [w1416]
      tunnel: w876 -> [w1417]
      tunnel: w875 -> [w1418]
      tunnel: [w1418] -> w1023
      tunnel: [w1417] -> w1022
      tunnel: [w1416] -> w1021
      tunnel: [w1415] -> w1020
      tunnel: [w1421] -> w638
      tunnel: [w1424] -> w871
      tunnel: [w1423] -> w872
      tunnel: [w1422] -> w812
      tunnel: w1023 -> [w1427]
      tunnel: w1022 -> [w1426]
      tunnel: w1021 -> [w1425]
      tunnel: w1020 -> [w1420]
      tunnel: [w1419] -> w682
      frame #0 {
        # "Write Data"
        n184 = To Single Precision Float(number="Capacitance (uF)") -> (single precision float=w1414:sgl)
        n185 = To Variant(anything=w1414) -> (Variant=w1415:variant)
      }
      frame #1 {
        # "Resolve To TC"
        n186 = call <userlib>:"Resolve To TC Type.vi"("Handle"=w1425, "TypHdl"=w1426, "WData"=w1420, "error in"=w1427) -> ("Handle"=w1423:u32, "TypHdl"=w1424:u32, "bHasMatched"=w1419:bool, "ADSWData"=w1422:variant, "error out"=w1421:errorcluster)  [unwired: 7 in]
      }
    }
    n187 = flat-sequence {
      tunnel: w853 -> [w1386]
      tunnel: w852 -> [w1387]
      tunnel: w851 -> [w1388]
      tunnel: [w1388] -> w1015
      tunnel: [w1387] -> w1014
      tunnel: [w1386] -> w1013
      tunnel: [w1385] -> w1012
      tunnel: w742 -> [w1383]
      tunnel: [w1391] -> w632
      tunnel: [w1394] -> w847
      tunnel: [w1393] -> w848
      tunnel: [w1392] -> w810
      tunnel: w1015 -> [w1397]
      tunnel: w1014 -> [w1396]
      tunnel: w1013 -> [w1395]
      tunnel: w1012 -> [w1390]
      tunnel: [w1389] -> w686
      frame #0 {
        # "Write Data"
        n188 = To Long Integer(number=w1383) -> (32bit integer=w1384:i32)
        n189 = To Variant(anything=w1384) -> (Variant=w1385:variant)
      }
      frame #1 {
        # "Resolve To TC"
        n190 = call <userlib>:"Resolve To TC Type.vi"("Handle"=w1395, "TypHdl"=w1396, "WData"=w1390, "error in"=w1397) -> ("Handle"=w1393:u32, "TypHdl"=w1394:u32, "bHasMatched"=w1389:bool, "ADSWData"=w1392:variant, "error out"=w1391:errorcluster)  [unwired: 7 in]
      }
    }
    n191 = flat-sequence {
      tunnel: w885 -> [w1432]
      tunnel: [w1430] -> _
      tunnel: w883 -> [w1433]
      tunnel: [w1433] -> w1027
      tunnel: [w1430] -> w1026
      tunnel: [w1432] -> w1025
      tunnel: [w1431] -> w1024
      tunnel: w884 -> [w1430]
      tunnel: [w1436] -> w641
      tunnel: [w1439] -> w887
      tunnel: [w1438] -> w886
      tunnel: [w1437] -> w813
      tunnel: w1027 -> [w1442]
      tunnel: w1026 -> [w1441]
      tunnel: w1025 -> [w1440]
      tunnel: w1024 -> [w1435]
      tunnel: [w1434] -> w680
      frame #0 {
        # "Write Data"
        n192 = To Long Integer(number="Cycle Time (Sec)") -> (32bit integer=w1429:i32)
        n193 = To Variant(anything=w1429) -> (Variant=w1431:variant)
      }
      frame #1 {
        # "Resolve To TC"
        n194 = call <userlib>:"Resolve To TC Type.vi"("Handle"=w1440, "TypHdl"=w1441, "WData"=w1435, "error in"=w1442) -> ("Handle"=w1438:u32, "TypHdl"=w1439:u32, "bHasMatched"=w1434:bool, "ADSWData"=w1437:variant, "error out"=w1436:errorcluster)  [unwired: 7 in]
      }
    }
    n195 = flat-sequence {
      tunnel: w865 -> [w1401]
      tunnel: w864 -> [w1402]
      tunnel: w863 -> [w1403]
      tunnel: [w1403] -> w1019
      tunnel: [w1402] -> w1018
      tunnel: [w1401] -> w1017
      tunnel: [w1400] -> w1016
      tunnel: [w1406] -> w635
      tunnel: [w1409] -> w859
      tunnel: [w1408] -> w860
      tunnel: [w1407] -> w811
      tunnel: w1019 -> [w1412]
      tunnel: w1018 -> [w1411]
      tunnel: w1017 -> [w1410]
      tunnel: w1016 -> [w1405]
      tunnel: [w1404] -> w684
      frame #0 {
        # "Write Data"
        n196 = To Long Integer(number="Target Charge Volt (V) - Min 1500V - TEMPORARY LIMIT 12kV") -> (32bit integer=w1399:i32)
        n197 = To Variant(anything=w1399) -> (Variant=w1400:variant)
      }
      frame #1 {
        # "Resolve To TC"
        n198 = call <userlib>:"Resolve To TC Type.vi"("Handle"=w1410, "TypHdl"=w1411, "WData"=w1405, "error in"=w1412) -> ("Handle"=w1408:u32, "TypHdl"=w1409:u32, "bHasMatched"=w1404:bool, "ADSWData"=w1407:variant, "error out"=w1406:errorcluster)  [unwired: 7 in]
      }
    }
    n199 = flat-sequence {
      tunnel: w841 -> [w1371]
      tunnel: w840 -> [w1372]
      tunnel: w839 -> [w1373]
      tunnel: [w1373] -> w1011
      tunnel: [w1372] -> w1010
      tunnel: [w1371] -> w1009
      tunnel: [w1370] -> w1008
      tunnel: [w1376] -> w629
      tunnel: [w1379] -> w835
      tunnel: [w1378] -> w836
      tunnel: [w1377] -> w809
      tunnel: w1011 -> [w1382]
      tunnel: w1010 -> [w1381]
      tunnel: w1009 -> [w1380]
      tunnel: w1008 -> [w1375]
      tunnel: [w1374] -> w688
      frame #0 {
        # "Write Data"
        n200 = To Single Precision Float(number="Hold Time Before Shot (seconds)") -> (single precision float=w1369:sgl)
        n201 = To Variant(anything=w1369) -> (Variant=w1370:variant)
      }
      frame #1 {
        # "Resolve To TC"
        n202 = call <userlib>:"Resolve To TC Type.vi"("Handle"=w1380, "TypHdl"=w1381, "WData"=w1375, "error in"=w1382) -> ("Handle"=w1378:u32, "TypHdl"=w1379:u32, "bHasMatched"=w1374:bool, "ADSWData"=w1377:variant, "error out"=w1376:errorcluster)  [unwired: 7 in]
      }
    }
    n203 = To Word Integer(number="Cap 1 Fault Temp (Cel)") -> (16bit integer=w466:i16)
    n204 = flat-sequence {
      tunnel: w901 -> [w1281]
      tunnel: w900 -> [w1282]
      tunnel: w899 -> [w1283]
      tunnel: [w1283] -> w987
      tunnel: [w1282] -> w986
      tunnel: [w1281] -> w985
      tunnel: [w1280] -> w984
      tunnel: [w1286] -> w643
      tunnel: [w1289] -> w895
      tunnel: [w1288] -> w896
      tunnel: [w1287] -> w814
      tunnel: w987 -> [w1292]
      tunnel: w986 -> [w1291]
      tunnel: w985 -> [w1290]
      tunnel: w984 -> [w1285]
      tunnel: [w1284] -> w679
      frame #0 {
        # "Write Data"
        n205 = And(x="CLEAR FAULT", y="CLEAR FAULT") -> (x .and. y?=w1279:bool)
        n206 = To Variant(anything=w1279) -> (Variant=w1280:variant)
      }
      frame #1 {
        # "Resolve To TC"
        n207 = call <userlib>:"Resolve To TC Type.vi"("Handle"=w1290, "TypHdl"=w1291, "WData"=w1285, "error in"=w1292) -> ("Handle"=w1288:u32, "TypHdl"=w1289:u32, "bHasMatched"=w1284:bool, "ADSWData"=w1287:variant, "error out"=w1286:errorcluster)  [unwired: 7 in]
      }
    }
    n208 = flat-sequence {
      tunnel: w949 -> [w1341]
      tunnel: w948 -> [w1342]
      tunnel: w947 -> [w1343]
      tunnel: [w1343] -> w1003
      tunnel: [w1342] -> w1002
      tunnel: [w1341] -> w1001
      tunnel: [w1340] -> w1000
      tunnel: [w1346] -> w655
      tunnel: [w1349] -> w943
      tunnel: [w1348] -> w944
      tunnel: [w1347] -> w818
      tunnel: w1003 -> [w1352]
      tunnel: w1002 -> [w1351]
      tunnel: w1001 -> [w1350]
      tunnel: w1000 -> [w1345]
      tunnel: [w1344] -> w671
      frame #0 {
        # "Write Data"
        n209 = And(x="Hold", y="Hold") -> (x .and. y?=w1339:bool)
        n210 = To Variant(anything=w1339) -> (Variant=w1340:variant)
      }
      frame #1 {
        # "Resolve To TC"
        n211 = call <userlib>:"Resolve To TC Type.vi"("Handle"=w1350, "TypHdl"=w1351, "WData"=w1345, "error in"=w1352) -> ("Handle"=w1348:u32, "TypHdl"=w1349:u32, "bHasMatched"=w1344:bool, "ADSWData"=w1347:variant, "error out"=w1346:errorcluster)  [unwired: 7 in]
      }
    }
    n212 = flat-sequence {
      tunnel: w925 -> [w1311]
      tunnel: w924 -> [w1312]
      tunnel: w923 -> [w1313]
      tunnel: [w1313] -> w995
      tunnel: [w1312] -> w994
      tunnel: [w1311] -> w993
      tunnel: [w1310] -> w992
      tunnel: [w1316] -> w649
      tunnel: [w1319] -> w919
      tunnel: [w1318] -> w920
      tunnel: [w1317] -> w816
      tunnel: w995 -> [w1322]
      tunnel: w994 -> [w1321]
      tunnel: w993 -> [w1320]
      tunnel: w992 -> [w1315]
      tunnel: [w1314] -> w675
      frame #0 {
        # "Write Data"
        n213 = And(x="Shot", y="Shot") -> (x .and. y?=w1309:bool)
        n214 = To Variant(anything=w1309) -> (Variant=w1310:variant)
      }
      frame #1 {
        # "Resolve To TC"
        n215 = call <userlib>:"Resolve To TC Type.vi"("Handle"=w1320, "TypHdl"=w1321, "WData"=w1315, "error in"=w1322) -> ("Handle"=w1318:u32, "TypHdl"=w1319:u32, "bHasMatched"=w1314:bool, "ADSWData"=w1317:variant, "error out"=w1316:errorcluster)  [unwired: 7 in]
      }
    }
    n216 = flat-sequence {
      tunnel: w957 -> [w1357]
      tunnel: [w1353] -> _
      tunnel: w955 -> [w1358]
      tunnel: [w1358] -> w1007
      tunnel: [w1353] -> w1006
      tunnel: [w1357] -> w1005
      tunnel: [w1356] -> w1004
      tunnel: w956 -> [w1353]
      tunnel: [w1361] -> w658
      tunnel: [w1364] -> w959
      tunnel: [w1363] -> w958
      tunnel: [w1362] -> w819
      tunnel: w1007 -> [w1367]
      tunnel: w1006 -> [w1366]
      tunnel: w1005 -> [w1365]
      tunnel: w1004 -> [w1360]
      tunnel: [w1359] -> w669
      frame #0 {
        # "Write Data"
        n217 = And(x="Manual/Auto", y="Manual/Auto") -> (x .and. y?=w1355:bool)
        n218 = To Variant(anything=w1355) -> (Variant=w1356:variant)
      }
      frame #1 {
        # "Resolve To TC"
        n219 = call <userlib>:"Resolve To TC Type.vi"("Handle"=w1365, "TypHdl"=w1366, "WData"=w1360, "error in"=w1367) -> ("Handle"=w1363:u32, "TypHdl"=w1364:u32, "bHasMatched"=w1359:bool, "ADSWData"=w1362:variant, "error out"=w1361:errorcluster)  [unwired: 7 in]
      }
    }
    n220 = flat-sequence {
      tunnel: w937 -> [w1326]
      tunnel: w936 -> [w1327]
      tunnel: w935 -> [w1328]
      tunnel: [w1328] -> w999
      tunnel: [w1327] -> w998
      tunnel: [w1326] -> w997
      tunnel: [w1325] -> w996
      tunnel: [w1331] -> w652
      tunnel: [w1334] -> w931
      tunnel: [w1333] -> w932
      tunnel: [w1332] -> w817
      tunnel: w999 -> [w1337]
      tunnel: w998 -> [w1336]
      tunnel: w997 -> [w1335]
      tunnel: w996 -> [w1330]
      tunnel: [w1329] -> w673
      frame #0 {
        # "Write Data"
        n221 = And(x="Charge", y="Charge") -> (x .and. y?=w1324:bool)
        n222 = To Variant(anything=w1324) -> (Variant=w1325:variant)
      }
      frame #1 {
        # "Resolve To TC"
        n223 = call <userlib>:"Resolve To TC Type.vi"("Handle"=w1335, "TypHdl"=w1336, "WData"=w1330, "error in"=w1337) -> ("Handle"=w1333:u32, "TypHdl"=w1334:u32, "bHasMatched"=w1329:bool, "ADSWData"=w1332:variant, "error out"=w1331:errorcluster)  [unwired: 7 in]
      }
    }
    n224 = flat-sequence {
      tunnel: w913 -> [w1296]
      tunnel: w912 -> [w1297]
      tunnel: w911 -> [w1298]
      tunnel: [w1298] -> w991
      tunnel: [w1297] -> w990
      tunnel: [w1296] -> w989
      tunnel: [w1295] -> w988
      tunnel: [w1301] -> w646
      tunnel: [w1304] -> w907
      tunnel: [w1303] -> w908
      tunnel: [w1302] -> w815
      tunnel: w991 -> [w1307]
      tunnel: w990 -> [w1306]
      tunnel: w989 -> [w1305]
      tunnel: w988 -> [w1300]
      tunnel: [w1299] -> w677
      frame #0 {
        # "Write Data"
        n225 = And(x="HV Switch Mode", y="HV Switch Mode") -> (x .and. y?=w1294:bool)
        n226 = To Variant(anything=w1294) -> (Variant=w1295:variant)
      }
      frame #1 {
        # "Resolve To TC"
        n227 = call <userlib>:"Resolve To TC Type.vi"("Handle"=w1305, "TypHdl"=w1306, "WData"=w1300, "error in"=w1307) -> ("Handle"=w1303:u32, "TypHdl"=w1304:u32, "bHasMatched"=w1299:bool, "ADSWData"=w1302:variant, "error out"=w1301:errorcluster)  [unwired: 7 in]
      }
    }
    n228 = flat-sequence {
      tunnel: w973 -> [w1242]
      tunnel: w972 -> [w1243]
      tunnel: w971 -> [w1244]
      tunnel: [w1244] -> w733
      tunnel: [w1243] -> w732
      tunnel: [w1242] -> w731
      tunnel: [w1241] -> w730
      tunnel: w733 -> [w1253]
      tunnel: w732 -> [w1252]
      tunnel: w731 -> [w1251]
      tunnel: w730 -> [w1246]
      tunnel: [w1247] -> w661
      tunnel: [w1250] -> w967
      tunnel: [w1249] -> w968
      tunnel: [w1248] -> w729
      tunnel: [w1245] -> w667
      frame #0 {
        # "Write Data"
        n229 = And(x="STOP", y="STOP") -> (x .and. y?=w1240:bool)
        n230 = To Variant(anything=w1240) -> (Variant=w1241:variant)
      }
      frame #1 {
        # "Resolve To TC"
        n231 = call <userlib>:"Resolve To TC Type.vi"("Handle"=w1251, "TypHdl"=w1252, "WData"=w1246, "error in"=w1253) -> ("Handle"=w1249:u32, "TypHdl"=w1250:u32, "bHasMatched"=w1245:bool, "ADSWData"=w1248:variant, "error out"=w1247:errorcluster)  [unwired: 7 in]
      }
    }
    n232 = flat-sequence {
      tunnel: w617 -> [w1189]
      tunnel: w616 -> [w1185]
      tunnel: w615 -> [w1190]
      tunnel: [w1190] -> w626
      tunnel: [w1185] -> w625
      tunnel: [w1189] -> w624
      tunnel: [w1188] -> w623
      tunnel: [w1193] -> w468
      tunnel: [w1196] -> w610
      tunnel: [w1195] -> w611
      tunnel: [w1194] -> w614
      tunnel: w626 -> [w1199]
      tunnel: w625 -> [w1198]
      tunnel: w624 -> [w1197]
      tunnel: w623 -> [w1192]
      tunnel: [w1191] -> w608
      frame #0 {
        # "Write Data"
        n233 = And(x="Reset Test Number", y="Reset Test Number") -> (x .and. y?=w1187:bool)
        n234 = To Variant(anything=w1187) -> (Variant=w1188:variant)
      }
      frame #1 {
        # "Resolve To TC"
        n235 = call <userlib>:"Resolve To TC Type.vi"("Handle"=w1197, "TypHdl"=w1198, "WData"=w1192, "error in"=w1199) -> ("Handle"=w1195:u32, "TypHdl"=w1196:u32, "bHasMatched"=w1191:bool, "ADSWData"=w1194:variant, "error out"=w1193:errorcluster)  [unwired: 7 in]
      }
    }
    n236 = flat-sequence {
      tunnel: w983 -> [w1208]
      tunnel: w982 -> [w1209]
      tunnel: w979 -> [w1210]
      tunnel: [w1210] -> w728
      tunnel: [w1209] -> w727
      tunnel: [w1208] -> w726
      tunnel: [w1207] -> w725
      tunnel: [w1205] -> _
      tunnel: [w1205] -> w724
      tunnel: w741 -> [w1205]
      tunnel: w740 -> [w1204]
      tunnel: [w1204] -> w723
      tunnel: w739 -> [w1203]
      tunnel: [w1203] -> w722
      tunnel: w738 -> [w1202]
      tunnel: [w1202] -> w721
      tunnel: w737 -> [w1201]
      tunnel: [w1201] -> w720
      tunnel: ["START"] -> w551
      tunnel: w728 -> [w1224]
      tunnel: w727 -> [w1223]
      tunnel: w726 -> [w1222]
      tunnel: w725 -> [w1217]
      tunnel: [w1218] -> w719
      tunnel: [w1221] -> w718
      tunnel: [w1220] -> w717
      tunnel: [w1219] -> w716
      tunnel: [w1216] -> w715
      tunnel: w724 -> [w1215]
      tunnel: [w1215] -> w714
      tunnel: w723 -> [w1214]
      tunnel: [w1214] -> w713
      tunnel: w722 -> [w1213]
      tunnel: [w1213] -> w712
      tunnel: w721 -> [w1212]
      tunnel: [w1212] -> w711
      tunnel: [w1211] -> w710
      tunnel: w720 -> [w1211]
      tunnel: [w1235] -> w693
      tunnel: [w1236] -> w981
      tunnel: [w1237] -> w980
      tunnel: [w1238] -> w664
      tunnel: w719 -> [w1238]
      tunnel: w718 -> [w1237]
      tunnel: w717 -> [w1236]
      tunnel: w716 -> [w1227]
      tunnel: w715 -> [w1235]
      tunnel: w714 -> [w1234]
      tunnel: w713 -> [w1233]
      tunnel: w712 -> [w1232]
      tunnel: w711 -> [w1231]
      tunnel: w710 -> [w1230]
      tunnel: [w1229] -> w736
      tunnel: [w1228] -> w735
      tunnel: [w1226] -> w665
      tunnel: [w1225] -> w708
      frame #0 {
        # "Write Data"
        n237 = And(x="START", y="START") -> (x .and. y?=w1206:bool)
        n238 = To Variant(anything=w1206) -> (Variant=w1207:variant)
      }
      frame #1 {
        # "Resolve To TC"
        n239 = call <userlib>:"Resolve To TC Type.vi"("Handle"=w1222, "TypHdl"=w1223, "WData"=w1217, "error in"=w1224) -> ("Handle"=w1220:u32, "TypHdl"=w1221:u32, "bHasMatched"=w1216:bool, "ADSWData"=w1219:variant, "error out"=w1218:errorcluster)  [unwired: 7 in]
      }
      frame #2 {
        # "Write"
        n240 = call <userlib>:"Send Writer-Request.vi"("Handle"=w1234, "SymbolName"=w1233, "WriterMode"=w1232, "WriteHandle"=w1231, "error constant"=w1230, "ADS Write Data"=w1227) -> ("Handle"=w1229:u32, "WriteHandle"=w1228:u32, "Write status?"=w1225:bool, "error IO"=w1226:errorcluster)  [unwired: 5 in, 1 out]
      }
    }
    n241 = To Variant(anything=w466) -> (Variant=w465:variant)
    n242 = call-poly <userlib>:"Write TypeResolved.vi"("Handle"=w446, "SymbolName"=w456, "WData"=w457, "error constant"=w455) -> ("Write Status?"=w451:bool, "Has Matched?"=w452:bool, "error out"=w454:errorcluster)  [unwired: 8 in, 1 out]
    n243 = call-poly <userlib>:"Write TypeResolved.vi"("Handle"=w446, "SymbolName"=w463, "WData"=w465, "error constant"=w464) -> ("Write Status?"=w460:bool, "Has Matched?"=w462:bool, "error out"=w461:errorcluster)  [unwired: 8 in, 1 out]
    n244 = To Single Precision Float(number="Duty Cycle") -> (single precision float=w510:sgl)
    n245 = And(x="Voltage Held by PSU", y="Voltage Held by PSU") -> (x .and. y?=w498:bool)
    n246 = And(x="Current Control", y="Current Control") -> (x .and. y?=w517:bool)
    n247 = To Variant(anything=w510) -> (Variant=w514:variant)
    n248 = And(x="Dump", y="Dump") -> (x .and. y?=w526:bool)
    n249 = To Variant(anything=w498) -> (Variant=w496:variant)
    n250 = To Variant(anything=w517) -> (Variant=w515:variant)
    n251 = To Variant(anything=w526) -> (Variant=w527:variant)
    n252 = call-poly <userlib>:"Write TypeResolved.vi"("Handle"=w446, "SymbolName"=w499, "WData"=w496, "error constant"=w495) -> ("Write Status?"=w488:bool, "Has Matched?"=w489:bool, "error out"=w494:errorcluster)  [unwired: 8 in, 1 out]
    n253 = flat-sequence {
      tunnel: w834 -> [w1578]
      tunnel: w833 -> [w1576]
      tunnel: w832 -> [w1574]
      tunnel: [w1577] -> w1062
      tunnel: [w1575] -> w1061
      tunnel: [w1573] -> w1060
      tunnel: [w1572] -> w1059
      tunnel: [w1571] -> w1058
      tunnel: [w1570] -> w1057
      tunnel: [w1569] -> w1056
      tunnel: [w1568] -> w1055
      tunnel: [w1567] -> w1054
      tunnel: [w1566] -> w1053
      tunnel: [w1565] -> w1052
      tunnel: w830 -> [w1564]
      tunnel: w829 -> [w1563]
      tunnel: w828 -> [w1562]
      tunnel: w827 -> [w1561]
      tunnel: w826 -> [w1560]
      tunnel: w825 -> [w1559]
      tunnel: [w1558] -> w1051
      tunnel: [w1557] -> w1050
      tunnel: [w1556] -> w1049
      tunnel: [w1555] -> w1048
      tunnel: [w1554] -> w1047
      tunnel: [w1553] -> w1046
      tunnel: [w1552] -> w1045
      tunnel: [w1551] -> w1044
      tunnel: [w1550] -> w1043
      tunnel: [w1549] -> w1042
      tunnel: [w1548] -> w1041
      tunnel: [w1547] -> w1040
      tunnel: [w1546] -> w1039
      tunnel: [w1545] -> w1038
      tunnel: [w1544] -> w1037
      tunnel: [w1543] -> w1036
      tunnel: [w1542] -> w1035
      tunnel: [w1541] -> w1034
      tunnel: [w1540] -> w1033
      tunnel: [w1539] -> w1032
      tunnel: [w1538] -> w1031
      tunnel: [w1537] -> w1030
      tunnel: [w1536] -> w1029
      tunnel: [w1535] -> w1028
      tunnel: w792 -> [w1534]
      tunnel: [w1533] -> w791
      tunnel: [w1532] -> w790
      tunnel: [w1531] -> w789
      tunnel: [w1530] -> w788
      tunnel: [w1529] -> w787
      tunnel: w785 -> [w1447]
      tunnel: [w1528] -> w784
      tunnel: w782 -> [w1527]
      tunnel: [w1526] -> w781
      tunnel: [w1525] -> w780
      tunnel: [w1524] -> w779
      tunnel: w778 -> [w1523]
      tunnel: w777 -> [w1522]
      tunnel: [w1521] -> w776
      tunnel: [w1520] -> w775
      tunnel: [w1519] -> w774
      tunnel: [w1518] -> w773
      tunnel: [w1517] -> w772
      tunnel: [w1516] -> w771
      tunnel: [w1515] -> w770
      tunnel: [w1514] -> w769
      tunnel: w761 -> [w1513]
      tunnel: w760 -> [w1512]
      tunnel: w759 -> [w1511]
      tunnel: [w1510] -> w758
      tunnel: [w1509] -> w757
      tunnel: [w1508] -> w756
      tunnel: [w1507] -> w755
      tunnel: [w1506] -> w754
      tunnel: [w1505] -> w753
      tunnel: [w1504] -> w752
      tunnel: [w1503] -> w751
      tunnel: [w1502] -> w750
      tunnel: [w1501] -> w749
      tunnel: [w1500] -> w748
      tunnel: [w1499] -> w747
      tunnel: [w1443] -> _
      tunnel: w734 -> [w1443]
      tunnel: [w1498] -> w602
      tunnel: [w1497] -> w601
      tunnel: [w1496] -> w600
      tunnel: w599 -> [w1495]
      tunnel: [w1494] -> w595
      tunnel: w594 -> [w1493]
      tunnel: [w1492] -> w593
      tunnel: [w1491] -> w592
      tunnel: [w1490] -> w591
      tunnel: [w1489] -> w590
      tunnel: w589 -> [w1488]
      tunnel: w588 -> [w1487]
      tunnel: w587 -> [w1486]
      tunnel: [w1485] -> w586
      tunnel: [w1484] -> w585
      tunnel: [w1483] -> w583
      tunnel: [w1482] -> w581
      tunnel: [w1481] -> w580
      tunnel: [w1480] -> w579
      tunnel: [w1479] -> w578
      tunnel: [w1478] -> w575
      tunnel: w574 -> [w1477]
      tunnel: [w1476] -> w573
      tunnel: [w1475] -> w572
      tunnel: [w1474] -> w571
      tunnel: w549 -> [w1473]
      tunnel: w548 -> [w1472]
      tunnel: [w1471] -> w547
      tunnel: [w1470] -> w546
      tunnel: [w1469] -> w545
      tunnel: [w1468] -> w544
      tunnel: [w1467] -> w543
      tunnel: [w1466] -> w542
      tunnel: w541 -> [w1465]
      tunnel: [w1464] -> w540
      tunnel: [w1463] -> w539
      tunnel: [w1462] -> w538
      tunnel: w524 -> [w1461]
      tunnel: [w1460] -> w523
      tunnel: [w1459] -> w522
      tunnel: [w1458] -> w521
      tunnel: [w1457] -> w483
      tunnel: [w1456] -> w482
      tunnel: w481 -> [w1455]
      tunnel: w480 -> [w1453]
      tunnel: [w1454] -> w479
      tunnel: [w1452] -> w478
      tunnel: [w1451] -> w477
      tunnel: [w1450] -> w476
      tunnel: [w1449] -> w470
      tunnel: w438 -> [w1448]
      tunnel: [w1446] -> w437
      tunnel: [w1445] -> w436
      tunnel: [w1444] -> w435
      tunnel: w1062 -> [w1797]
      tunnel: w1061 -> [w1810]
      tunnel: w1060 -> [_]
      tunnel: w1059 -> [w1796]
      tunnel: w1058 -> [w1795]
      tunnel: w1057 -> [w1626]
      tunnel: [w1725] -> w831
      tunnel: w1056 -> [w1809]
      tunnel: w1055 -> [w1811]
      tunnel: w1054 -> [w1813]
      tunnel: w1053 -> [w1635]
      tunnel: w1052 -> [_]
      tunnel: w1051 -> [w1792]
      tunnel: w1050 -> [w1807]
      tunnel: w1049 -> [w1805]
      tunnel: w1048 -> [w1803]
      tunnel: w1047 -> [w1801]
      tunnel: w1046 -> [w1799]
      tunnel: [w1738] -> w824
      tunnel: w1045 -> [w1791]
      tunnel: w1044 -> [w1790]
      tunnel: w1043 -> [w1789]
      tunnel: w1042 -> [w1788]
      tunnel: w1041 -> [w1787]
      tunnel: w1040 -> [w1786]
      tunnel: w1039 -> [_]
      tunnel: w1038 -> [w1624]
      tunnel: w1037 -> [_]
      tunnel: w1036 -> [w1622]
      tunnel: w1035 -> [_]
      tunnel: w1034 -> [w1620]
      tunnel: w1033 -> [_]
      tunnel: w1032 -> [w1618]
      tunnel: w1031 -> [_]
      tunnel: w1030 -> [w1616]
      tunnel: w1029 -> [_]
      tunnel: w1028 -> [w1614]
      tunnel: [w1740] -> w823
      tunnel: [w1742] -> w822
      tunnel: [w1744] -> w821
      tunnel: [w1746] -> w820
      tunnel: w791 -> [w1612]
      tunnel: w790 -> [w1777]
      tunnel: w789 -> [_]
      tunnel: w788 -> [w1709]
      tunnel: w787 -> [w1773]
      tunnel: [w1729] -> w786
      tunnel: w784 -> [w1776]
      tunnel: [w1727] -> w783
      tunnel: w781 -> [w1775]
      tunnel: w780 -> [w1588]
      tunnel: w779 -> [_]
      tunnel: w776 -> [w1771]
      tunnel: w775 -> [w1770]
      tunnel: w774 -> [w1767]
      tunnel: w773 -> [w1766]
      tunnel: w772 -> [w1765]
      tunnel: w771 -> [w1764]
      tunnel: w770 -> [_]
      tunnel: w769 -> [_]
      tunnel: [w1731] -> w768
      tunnel: [w1733] -> w767
      tunnel: [w1748] -> w764
      tunnel: [w1751] -> w763
      tunnel: [w1750] -> w762
      tunnel: w758 -> [w1762]
      tunnel: w757 -> [w1760]
      tunnel: w756 -> [w1758]
      tunnel: w755 -> [w1630]
      tunnel: w754 -> [w1628]
      tunnel: w753 -> [w1632]
      tunnel: w752 -> [w1757]
      tunnel: w751 -> [w1756]
      tunnel: w750 -> [w1755]
      tunnel: w749 -> [_]
      tunnel: w748 -> [_]
      tunnel: w747 -> [_]
      tunnel: [w1736] -> w746
      tunnel: [w1734] -> w745
      tunnel: [w1723] -> w744
      tunnel: [w1724] -> w440
      tunnel: [w1715] -> w627
      tunnel: [w1717] -> w603
      tunnel: w602 -> [w1634]
      tunnel: w601 -> [w1720]
      tunnel: w600 -> [_]
      tunnel: [w1718] -> w598
      tunnel: w595 -> [w1712]
      tunnel: w593 -> [w1707]
      tunnel: w592 -> [w1704]
      tunnel: w591 -> [w1702]
      tunnel: w590 -> [w1689]
      tunnel: w586 -> [w1610]
      tunnel: w585 -> [w1701]
      tunnel: [w1700] -> w584
      tunnel: w583 -> [w1699]
      tunnel: [w1698] -> w582
      tunnel: w581 -> [w1697]
      tunnel: w580 -> [w1606]
      tunnel: w579 -> [w1696]
      tunnel: w578 -> [w1604]
      tunnel: [w1695] -> w577
      tunnel: [w1694] -> w576
      tunnel: w575 -> [w1608]
      tunnel: [w1693] -> w558
      tunnel: [w1692] -> w556
      tunnel: [w1691] -> w566
      tunnel: w573 -> [w1685]
      tunnel: w572 -> [w1602]
      tunnel: w571 -> [w1687]
      tunnel: [w1686] -> w570
      tunnel: w547 -> [w1681]
      tunnel: w546 -> [w1600]
      tunnel: w545 -> [w1683]
      tunnel: w544 -> [w1682]
      tunnel: w543 -> [w1677]
      tunnel: w542 -> [w1598]
      tunnel: w540 -> [w1663]
      tunnel: w539 -> [w1596]
      tunnel: w538 -> [w1676]
      tunnel: [w1669] -> w537
      tunnel: [w1668] -> w536
      tunnel: [w1667] -> w535
      tunnel: [w1666] -> w534
      tunnel: w523 -> [w1644]
      tunnel: w522 -> [w1661]
      tunnel: w521 -> [w1594]
      tunnel: [w1660] -> w520
      tunnel: w483 -> [w1592]
      tunnel: w482 -> [w1645]
      tunnel: w479 -> [w1640]
      tunnel: w478 -> [w1642]
      tunnel: w477 -> [w1641]
      tunnel: w476 -> [w1590]
      tunnel: [w1637] -> w475
      tunnel: [w1636] -> w474
      tunnel: w470 -> [_]
      tunnel: w437 -> [w1580]
      tunnel: w436 -> [w1585]
      tunnel: w435 -> [w1584]
      tunnel: [w1581] -> w434
      frame #0 {
        # "Read and Resolve Data."
        # "Read/Resolve Symbol N"
        # "Read Data and Resolve Type"
        n254 = call-poly <userlib>:"Read TypeResolved.vi"("Handle"=w1443, "SymbolName"=w1522, "error constant"=w1447) -> ("Handle"=w1515:u32, "Read Status?"=w1520:bool, "RData"=w1516:variant, "error out"=w1519:errorcluster)  [unwired: 9 in]
        n255 = call-poly <userlib>:"Read TypeResolved.vi"("Handle"=w1443, "SymbolName"=w1523, "error constant"=w1447) -> ("Handle"=w1514:u32, "Read Status?"=w1521:bool, "RData"=w1517:variant, "error out"=w1518:errorcluster)  [unwired: 9 in]
        n256 = call-poly <userlib>:"Read TypeResolved.vi"("Handle"=w1443, "SymbolName"=w1576, "error constant"=w1447) -> ("Handle"=w1566:u32, "Read Status?"=w1568:bool, "RData"=w1572:variant, "error out"=w1577:errorcluster)  [unwired: 9 in]
        n257 = call-poly <userlib>:"Read TypeResolved.vi"("Handle"=w1443, "SymbolName"=w1527, "error constant"=w1447) -> ("Handle"=w1524:u32, "Read Status?"=w1526:bool, "RData"=w1525:variant, "error out"=w1529:errorcluster)  [unwired: 9 in]
        n258 = call-poly <userlib>:"Read TypeResolved.vi"("Handle"=w1443, "SymbolName"=w1578, "error constant"=w1447) -> ("Handle"=w1565:u32, "Read Status?"=w1567:bool, "RData"=w1571:variant, "error out"=w1528:errorcluster)  [unwired: 9 in]
        n259 = call-poly <userlib>:"Read TypeResolved.vi"("Handle"=w1443, "SymbolName"=w1455, "error constant"=w1447) -> ("Read Status?"=w1454:bool, "RData"=w1457:variant, "error out"=w1456:errorcluster)  [unwired: 9 in, 1 out]
        n260 = call-poly <userlib>:"Read TypeResolved.vi"("Handle"=w1443, "SymbolName"=w1574, "error constant"=w1447) -> ("Handle"=w1573:u32, "Read Status?"=w1569:bool, "RData"=w1570:variant, "error out"=w1575:errorcluster)  [unwired: 9 in]
        n261 = call-poly <userlib>:"Read TypeResolved.vi"("Handle"=w1443, "SymbolName"=w1448, "error constant"=w1447) -> ("Read Status?"=w1444:bool, "RData"=w1446:variant, "error out"=w1445:errorcluster)  [unwired: 9 in, 1 out]
        n262 = call-poly <userlib>:"Read TypeResolved.vi"("Handle"=w1443, "SymbolName"=w1564, "error constant"=w1447) -> ("Handle"=w1546:u32, "Read Status?"=w1553:bool, "RData"=w1545:variant, "error out"=w1552:errorcluster)  [unwired: 9 in]
        n263 = call-poly <userlib>:"Read TypeResolved.vi"("Handle"=w1443, "SymbolName"=w1465, "error constant"=w1447) -> ("Read Status?"=w1464:bool, "RData"=w1463:variant, "error out"=w1462:errorcluster)  [unwired: 9 in, 1 out]
        n264 = call-poly <userlib>:"Read TypeResolved.vi"("Handle"=w1443, "SymbolName"=w1453, "error constant"=w1447) -> ("Read Status?"=w1451:bool, "RData"=w1450:variant, "error out"=w1452:errorcluster)  [unwired: 9 in, 1 out]
        n265 = call-poly <userlib>:"Read TypeResolved.vi"("Handle"=w1443, "SymbolName"=w1461, "error constant"=w1447) -> ("Read Status?"=w1460:bool, "RData"=w1458:variant, "error out"=w1459:errorcluster)  [unwired: 9 in, 1 out]
        n266 = call-poly <userlib>:"Read TypeResolved.vi"("Handle"=w1443, "SymbolName"=w1562, "error constant"=w1447) -> ("Handle"=w1542:u32, "Read Status?"=w1555:bool, "RData"=w1541:variant, "error out"=w1550:errorcluster)  [unwired: 9 in]
        n267 = call-poly <userlib>:"Read TypeResolved.vi"("Handle"=w1443, "SymbolName"=w1560, "error constant"=w1447) -> ("Handle"=w1538:u32, "Read Status?"=w1557:bool, "RData"=w1537:variant, "error out"=w1548:errorcluster)  [unwired: 9 in]
        n268 = call-poly <userlib>:"Read TypeResolved.vi"("Handle"=w1443, "SymbolName"=w1477, "error constant"=w1447) -> ("Read Status?"=w1476:bool, "RData"=w1475:variant, "error out"=w1474:errorcluster)  [unwired: 9 in, 1 out]
        n269 = call-poly <userlib>:"Read TypeResolved.vi"("Handle"=w1443, "SymbolName"=w1473, "error constant"=w1447) -> ("Read Status?"=w1471:bool, "RData"=w1470:variant, "error out"=w1469:errorcluster)  [unwired: 9 in, 1 out]
        n270 = call-poly <userlib>:"Read TypeResolved.vi"("Handle"=w1443, "SymbolName"=w1472, "error constant"=w1447) -> ("Read Status?"=w1467:bool, "RData"=w1466:variant, "error out"=w1468:errorcluster)  [unwired: 9 in, 1 out]
        n271 = call-poly <userlib>:"Read TypeResolved.vi"("Handle"=w1443, "SymbolName"=w1563, "error constant"=w1447) -> ("Handle"=w1544:u32, "Read Status?"=w1554:bool, "RData"=w1543:variant, "error out"=w1551:errorcluster)  [unwired: 9 in]
        n272 = call-poly <userlib>:"Read TypeResolved.vi"("Handle"=w1443, "SymbolName"=w1561, "error constant"=w1447) -> ("Handle"=w1540:u32, "Read Status?"=w1556:bool, "RData"=w1539:variant, "error out"=w1549:errorcluster)  [unwired: 9 in]
        n273 = call-poly <userlib>:"Read TypeResolved.vi"("Handle"=w1443, "SymbolName"=w1559, "error constant"=w1447) -> ("Handle"=w1536:u32, "Read Status?"=w1558:bool, "RData"=w1535:variant, "error out"=w1547:errorcluster)  [unwired: 9 in]
        n274 = call-poly <userlib>:"Read TypeResolved.vi"("Handle"=w1443, "SymbolName"=w1534, "error constant"=w1447) -> ("Handle"=w1531:u32, "Read Status?"=w1530:bool, "RData"=w1533:variant, "error out"=w1532:errorcluster)  [unwired: 9 in]
        n275 = call-poly <userlib>:"Read TypeResolved.vi"("Handle"=w1443, "SymbolName"=w1493, "error constant"=w1447) -> ("Handle"=w1449:u32, "Read Status?"=w1492:bool, "RData"=w1485:variant, "error out"=w1484:errorcluster)  [unwired: 9 in]
        n276 = call-poly <userlib>:"Read TypeResolved.vi"("Handle"=w1443, "SymbolName"=w1488, "error constant"=w1447) -> ("Read Status?"=w1491:bool, "RData"=w1478:variant, "error out"=w1483:errorcluster)  [unwired: 9 in, 1 out]
        n277 = call-poly <userlib>:"Read TypeResolved.vi"("Handle"=w1443, "SymbolName"=w1486, "error constant"=w1447) -> ("Read Status?"=w1489:bool, "RData"=w1479:variant, "error out"=w1480:errorcluster)  [unwired: 9 in, 1 out]
        n278 = call-poly <userlib>:"Read TypeResolved.vi"("Handle"=w1443, "SymbolName"=w1487, "error constant"=w1447) -> ("Read Status?"=w1490:bool, "RData"=w1481:variant, "error out"=w1482:errorcluster)  [unwired: 9 in, 1 out]
        n279 = call-poly <userlib>:"Read TypeResolved.vi"("Handle"=w1443, "SymbolName"=w1513, "error constant"=w1447) -> ("Handle"=w1501:u32, "Read Status?"=w1510:bool, "RData"=w1506:variant, "error out"=w1502:errorcluster)  [unwired: 9 in]
        n280 = call-poly <userlib>:"Read TypeResolved.vi"("Handle"=w1443, "SymbolName"=w1512, "error constant"=w1447) -> ("Handle"=w1500:u32, "Read Status?"=w1509:bool, "RData"=w1507:variant, "error out"=w1503:errorcluster)  [unwired: 9 in]
        n281 = call-poly <userlib>:"Read TypeResolved.vi"("Handle"=w1443, "SymbolName"=w1495, "error constant"=w1447) -> ("Handle"=w1496:u32, "Read Status?"=w1494:bool, "RData"=w1498:variant, "error out"=w1497:errorcluster)  [unwired: 9 in]
        n282 = call-poly <userlib>:"Read TypeResolved.vi"("Handle"=w1443, "SymbolName"=w1511, "error constant"=w1447) -> ("Handle"=w1499:u32, "Read Status?"=w1508:bool, "RData"=w1505:variant, "error out"=w1504:errorcluster)  [unwired: 9 in]
      }
      frame #1 {
        # "Cast Symbol N to LabVIEW Type"
        # "Variant To Data"
        n283 = To Variant(anything=w1590) -> (Variant=w1589:variant)
        n284 = To Variant(anything=w1632) -> (Variant=w1631:variant)
        n285 = To Variant(anything=w1604) -> (Variant=w1603:variant)
        n286 = To Variant(anything=w1630) -> (Variant=w1629:variant)
        n287 = To Variant(anything=w1598) -> (Variant=w1597:variant)
        n288 = To Variant(anything=w1600) -> (Variant=w1599:variant)
        n289 = To Variant(anything=w1592) -> (Variant=w1591:variant)
        n290 = To Variant(anything=w1602) -> (Variant=w1601:variant)
        n291 = To Variant(anything=w1594) -> (Variant=w1593:variant)
        n292 = To Variant(anything=w1596) -> (Variant=w1595:variant)
        n293 = To Variant(anything=w1628) -> (Variant=w1627:variant)
        n294 = To Variant(anything=w1612) -> (Variant=w1611:variant)
        n295 = To Variant(anything=w1610) -> (Variant=w1609:variant)
        n296 = To Variant(anything=w1608) -> (Variant=w1607:variant)
        n297 = To Variant(anything=w1622) -> (Variant=w1621:variant)
        n298 = To Variant(anything=w1588) -> (Variant=w1587:variant)
        n299 = To Variant(anything=w1606) -> (Variant=w1605:variant)
        n300 = To Variant(anything=w1626) -> (Variant=w1625:variant)
        n301 = To Variant(anything=w1624) -> (Variant=w1623:variant)
        n302 = To Variant(anything=w1614) -> (Variant=w1613:variant)
        n303 = To Variant(anything=w1634) -> (Variant=w1633:variant)
        n304 = To Variant(anything=w1620) -> (Variant=w1619:variant)
        n305 = To Variant(anything=w1616) -> (Variant=w1615:variant)
        n306 = To Variant(anything=w1618) -> (Variant=w1617:variant)
        n307 = Variant To Data(error in=w1585, Variant=w1580) -> (data=→"Spark Gap Voltage":i16, error out=w1581:errorcluster)  [unwired: 1 in]
        n308 = And(x=w1640, y=w1641) -> (x .and. y?=w1583:bool)
        n309 = Variant To Data(error in=w1645, Variant=w1591) -> (data=→"Test Interval (Sec)":i32, error out=w1637:errorcluster)  [unwired: 1 in]
        n310 = Variant To Data(error in=w1642, Variant=w1589) -> (data=→"Test Interval Fault":bool, error out=w1636:errorcluster)  [unwired: 1 in]
        n311 = And(x=w1583, y=w1584) -> (x .and. y?=w1582:bool)
        n312 = And(x=w1644, y=w1582) -> (x .and. y?=w1643:bool)
        n313 = And(x=w1663, y=w1643) -> (x .and. y?=w1662:bool)
        n314 = And(x=w1677, y=w1662) -> (x .and. y?=w1678:bool)
        n315 = And(x=w1681, y=w1678) -> (x .and. y?=w1680:bool)
        n316 = And(x=w1685, y=w1680) -> (x .and. y?=w1684:bool)
        n317 = And(x=w1689, y=w1684) -> (x .and. y?=w1688:bool)
        n318 = And(x=w1702, y=w1688) -> (x .and. y?=w1703:bool)
        n319 = And(x=w1704, y=w1703) -> (x .and. y?=w1705:bool)
        n320 = And(x=w1707, y=w1705) -> (x .and. y?=w1706:bool)
        n321 = And(x=w1709, y=w1706) -> (x .and. y?=w1708:bool)
        n322 = And(x=w1792, y=w1708) -> (x .and. y?=w1808:bool)
        n323 = And(x=w1807, y=w1808) -> (x .and. y?=w1806:bool)
        n324 = And(x=w1805, y=w1806) -> (x .and. y?=w1804:bool)
        n325 = And(x=w1803, y=w1804) -> (x .and. y?=w1802:bool)
        n326 = And(x=w1801, y=w1802) -> (x .and. y?=w1800:bool)
        n327 = And(x=w1799, y=w1800) -> (x .and. y?=w1798:bool)
        n328 = And(x=w1809, y=w1798) -> (x .and. y?=w1763:bool)
        n329 = And(x=w1762, y=w1763) -> (x .and. y?=w1761:bool)
        n330 = And(x=w1760, y=w1761) -> (x .and. y?=w1759:bool)
        n331 = And(x=w1758, y=w1759) -> (x .and. y?=w1711:bool)
        n332 = And(x=w1712, y=w1711) -> (x .and. y?=w1710:bool)
        n333 = And(x=w1770, y=w1710) -> (x .and. y?=w1769:bool)
        n334 = And(x=w1771, y=w1769) -> (x .and. y?=w1768:bool)
        n335 = And(x=w1775, y=w1768) -> (x .and. y?=w1774:bool)
        n336 = And(x=w1813, y=w1774) -> (x .and. y?=w1812:bool)
        n337 = Variant To Data(error in=w1720, Variant=w1633) -> (data=→"Cap 1 Voltage (HVPS)":i16, error out=w1718:errorcluster)  [unwired: 1 in]
        n338 = Variant To Data(error in=w1791, Variant=w1623) -> (data=→"Discharge Fault":bool, error out=w1740:errorcluster)  [unwired: 1 in]
        n339 = Variant To Data(error in=w1810, Variant=w1625) -> (data=→"Charge Fault":bool, error out=w1738:errorcluster)  [unwired: 1 in]
        n340 = Variant To Data(error in=w1789, Variant=w1619) -> (data=→"Cap 1 Temp\nExceeded Fault":bool, error out=w1744:errorcluster)  [unwired: 1 in]
        n341 = And(x=w1811, y=w1812) -> (x .and. y?=→"Read Status":bool)
        n342 = Variant To Data(error in=w1790, Variant=w1621) -> (data=→"Hold Fault":bool, error out=w1742:errorcluster)  [unwired: 1 in]
        n343 = Variant To Data(error in=w1757, Variant=w1631) -> (data=→"Load Temperature":i16, error out=w1723:errorcluster)  [unwired: 1 in]
        n344 = Variant To Data(error in=w1788, Variant=w1617) -> (data=→"Ambient Temp\nExceeded Fault":bool, error out=w1746:errorcluster)  [unwired: 1 in]
        n345 = Variant To Data(error in=w1787, Variant=w1615) -> (data=→"PSU Fault":bool, error out=w1748:errorcluster)  [unwired: 1 in]
        n346 = Variant To Data(error in=w1786, Variant=w1613) -> (data=→"Control Sys Fault":bool, error out=w1750:errorcluster)  [unwired: 1 in]
        n347 = Variant To Data(error in=w1777, Variant=w1611) -> (data=→"test Running":bool, error out=w1751:errorcluster)  [unwired: 1 in]
        n348 = Variant To Data(error in=w1755, Variant=w1627) -> (data=→"Ambient Temp":i16, error out=w1736:errorcluster)  [unwired: 1 in]
        n349 = Variant To Data(error in=w1696, Variant=w1603) -> (data=w1691:bool, error out=w1694:errorcluster)  [unwired: 1 in]
        "Soft Exception" <- w1691
        n350 = Variant To Data(error in=w1687, Variant=w1601) -> (data=w1586:bool, error out=w1669:errorcluster)  [unwired: 1 in]
        "EOC" <- w1586
        n351 = Variant To Data(error in=w1766, Variant=w1765) -> (data=w1675:i16, error out=w1731:errorcluster)  [unwired: 1 in]
        "Cap 1 Voltage" <- w1675
        n352 = Variant To Data(error in=w1756, Variant=w1629) -> (data=→"Soft Dump Temp":i16, error out=w1734:errorcluster)  [unwired: 1 in]
        n353 = Variant To Data(error in=w1701, Variant=w1609) -> (data=w1686:bool, error out=w1700:errorcluster)  [unwired: 1 in]
        "Softdump FB Fault" <- w1686
        n354 = Variant To Data(error in=w1697, Variant=w1605) -> (data=w1692:bool, error out=w1695:errorcluster)  [unwired: 1 in]
        "PSU HV FB Fault" <- w1692
        n355 = Variant To Data(error in=w1683, Variant=w1599) -> (data=w1657:bool, error out=w1668:errorcluster)  [unwired: 1 in]
        "SCR Ready" <- w1657
        n356 = Variant To Data(error in=w1682, Variant=w1597) -> (data=→"Maximum Test Number Reached":bool, error out=w1667:errorcluster)  [unwired: 1 in]
        n357 = Variant To Data(error in=w1699, Variant=w1607) -> (data=w1693:bool, error out=w1698:errorcluster)  [unwired: 1 in]
        "Charge FB Fault" <- w1693
        n358 = Variant To Data(error in=w1661, Variant=w1593) -> (data=w1658:bool, error out=w1660:errorcluster)  [unwired: 1 in]
        "Scope Trig" <- w1658
        n359 = Variant To Data(error in=w1773, Variant=w1587) -> (data=w1659:u8, error out=w1729:errorcluster)  [unwired: 1 in]
        "Process Step" <- w1659
        n360 = Variant To Data(error in=w1767, Variant=w1764) -> (data=→"Cap 1 Temperature":i16, error out=w1733:errorcluster)  [unwired: 1 in]
        n361 = Variant To Data(error in=w1676, Variant=w1595) -> (data=w1665:i16, error out=w1666:errorcluster)  [unwired: 1 in]
        "Expected Voltage" <- w1665
        n362 = Variant To Data(error in=w1797, Variant=w1796) -> (data=→"Estimated Charge Time (seconds)":sgl, error out=w1725:errorcluster)  [unwired: 1 in]
        n363 = To Double Precision Float(number=w1675) -> (double precision float=→"Waveform Chart - Capacitor Voltage (Probe, abs(Volts))":dbl)
        n364 = Variant To Data(error in=w1776, Variant=w1795) -> (data=→"Shot Number":i16, error out=w1727:errorcluster)  [unwired: 1 in]
        n365 = case shown="True" "Log Temperature Data" {
          tunnel: [errorcluster {"status"=FALSE, "code"=0, "source"=""} ("error out") w1824] -> w1717
          frame False {
          }
          frame True {
            n366 = local read "Cap 1 Temperature"() -> (w1825:i16)
            n367 = local read "test Running"() -> (w1823:bool)
            n368 = call "Write To Measurement File2"("Signals"=w1825, "Enable"=w1823, "Filename"="Capacitor Temperature Data Log File Path (.xlsx)") -> ("error out"=w1824:errorcluster)  [unwired: 14 in, 2 out]
          }
        }
        n369 = case shown="2" w1659 {
          tunnel: ["Charge" "Current Controlled Charge" "Hold - Ready for Shot" "Hold - Cap Open Circuited" "Shot" "Wait" "Dump" "Error" "Wait"] -> w1772
          tunnel: [TRUE TRUE TRUE TRUE TRUE TRUE FALSE FALSE FALSE] -> w1655
          tunnel: [FALSE ("Reset") FALSE ("Reset") FALSE ("Reset") FALSE ("Reset") TRUE ("Reset") FALSE ("Reset") FALSE ("Reset") TRUE ("Reset") FALSE ("Reset")] -> _
          frame 1 {
          }
          frame 6 {
          }
          frame 2 {
          }
          frame 7 {
          }
          frame 3 {
          }
          frame 4 {
          }
          frame 5 {
          }
          frame 99 {
          }
          frame 0, Default {
          }
        }
        "Test State" <- w1772
        n370 = local write "Scope Trig"(w1658) -> ()
        n371 = local read "Cap 1 Voltage"() -> (w1647:i16)
        n372 = case shown="True" "Log Capacitor Voltage" {
          tunnel: [errorcluster {"status"=FALSE, "code"=0, "source"=""} ("error out") w1821] -> w1715
          tunnel: w1675 -> [_ w1820]
          tunnel: w1655 -> [_ w1819]
          frame False {
          }
          frame True {
            n373 = local read "test Running"() -> (w1816:bool)
            n374 = And(x=w1819, y=w1816) -> (x .and. y?=w1817:bool)
            n375 = call "Write To Measurement File"("Signals"=w1820, "Enable"=w1817, "Filename"="Capacitor Voltage Data Log File Path (.xlsx)") -> ("error out"=w1821:errorcluster)  [unwired: 14 in, 2 out]
          }
        }
        n376 = Not(x=w1586) -> (.not. x?=w1673:bool)
        n377 = To Double Precision Float(number=w1647) -> (double precision float=w1671:dbl)
        n378 = To Double Precision Float(number=w1665) -> (double precision float=w1664:dbl)
        n379 = Boolean To (0,1)(Boolean=w1673) -> (0, 1=→"EOC":i16)
        n380 = Or(x=w1750, y=w1751) -> (x .or. y?=w1749:bool)
        n381 = Or(x=w1748, y=w1749) -> (x .or. y?=w1747:bool)
        n382 = Or(x=w1746, y=w1747) -> (x .or. y?=w1745:bool)
        n383 = Or(x=w1744, y=w1745) -> (x .or. y?=w1743:bool)
        n384 = Or(x=w1742, y=w1743) -> (x .or. y?=w1741:bool)
        n385 = Or(x=w1740, y=w1741) -> (x .or. y?=w1739:bool)
        n386 = Or(x=w1738, y=w1739) -> (x .or. y?=w1737:bool)
        n387 = Or(x=w1736, y=w1737) -> (x .or. y?=w1735:bool)
        n388 = Or(x=w1734, y=w1735) -> (x .or. y?=w1722:bool)
        n389 = Or(x=w1723, y=w1722) -> (x .or. y?=w1716:bool)
        n390 = Boolean To (0,1)(Boolean=w1657) -> (0, 1=→"SCR FB":i16)
        n391 = Bundle(w1671, w1664) -> (→"Capacitor Voltage":cluster{dbl, dbl})  [unwired: 1 in]
        n392 = local write "Process Step"(w1659) -> ()
        n393 = local read "Scope Trig"() -> (w1650:bool)
        n394 = local read "Test Interval (Sec)"() -> (w1653:i32)
        n395 = Not(x=w1650) -> (.not. x?=w1649:bool)
        n396 = call "Elapsed Time"("Time Target (s)"=w1653, "Reset"=w1649) -> ("Elapsed Time Text"=w1652:string)  [unwired: 10 in, 7 out]
        n397 = String Subset(string=w1652, offset (0)=2) -> (substring=→"Time Since Last Shot":string)  [unwired: 1 in]
        n398 = Or(x=w1717, y=w1716) -> (x .or. y?=w1714:bool)
        n399 = Or(x=w1715, y=w1714) -> (x .or. y?=w1713:bool)
        n400 = Or(x=w1733, y=w1713) -> (x .or. y?=w1732:bool)
        n401 = Or(x=w1731, y=w1732) -> (x .or. y?=w1730:bool)
        n402 = Or(x=w1729, y=w1730) -> (x .or. y?=w1728:bool)
        n403 = Or(x=w1727, y=w1728) -> (x .or. y?=w1726:bool)
        n404 = Or(x=w1725, y=w1726) -> (x .or. y?=w1724:bool)
        n405 = case shown="True" w1586 {
          frame False {
          }
          frame True {
            n406 = local write "Single"(TRUE) -> ()
          }
        }
        "Internal TwinCAT Handle ID Maps" <- w1635
      }
    }
    n407 = call-poly <userlib>:"Write TypeResolved.vi"("Handle"=w446, "SymbolName"=w518, "WData"=w514, "error constant"=w495) -> ("Write Status?"=w487:bool, "Has Matched?"=w490:bool, "error out"=w512:errorcluster)  [unwired: 8 in, 1 out]
    n408 = call-poly <userlib>:"Write TypeResolved.vi"("Handle"=w446, "SymbolName"=w519, "WData"=w515, "error constant"=w495) -> ("Write Status?"=w486:bool, "Has Matched?"=w491:bool, "error out"=w513:errorcluster)  [unwired: 8 in, 1 out]
    n409 = call <userlib>:"Send Writer-Request.vi"("Handle"=w978, "SymbolName"=w977, "WriterMode"=w976, "WriteHandle"=w975, "error constant"=w974, "ADS Write Data"=w729) -> ("Handle"=w970:u32, "WriteHandle"=w969:u32, "Write status?"=w707:bool, "error IO"=w662:errorcluster)  [unwired: 5 in, 1 out]
    n410 = call-poly <userlib>:"Write TypeResolved.vi"("Handle"=w446, "SymbolName"=w533, "WData"=w527, "error constant"=w532) -> ("Handle"=w528:u32, "Write Status?"=w485:bool, "Has Matched?"=w493:bool, "error out"=w529:errorcluster)  [unwired: 8 in]
    n411 = call <userlib>:"Send Writer-Request.vi"("Handle"=w894, "SymbolName"=w893, "WriterMode"=w892, "WriteHandle"=w890, "error constant"=w891, "ADS Write Data"=w813) -> ("Handle"=w889:u32, "WriteHandle"=w888:u32, "Write status?"=w509:bool, "error IO"=w642:errorcluster)  [unwired: 5 in, 1 out]
    n412 = call <userlib>:"Send Writer-Request.vi"("Handle"=w804, "SymbolName"=w803, "WriterMode"=w802, "WriteHandle"=w793, "error constant"=w801, "ADS Write Data"=w473) -> ("Handle"=w800:u32, "WriteHandle"=w799:u32, "Write status?"=w504:bool, "error IO"=w472:errorcluster)  [unwired: 5 in, 1 out]
    n413 = call <userlib>:"Send Writer-Request.vi"("Handle"=w882, "SymbolName"=w881, "WriterMode"=w880, "WriteHandle"=w879, "error constant"=w878, "ADS Write Data"=w812) -> ("Handle"=w874:u32, "WriteHandle"=w873:u32, "Write status?"=w508:bool, "error IO"=w639:errorcluster)  [unwired: 5 in, 1 out]
    n414 = call <userlib>:"Send Writer-Request.vi"("Handle"=w858, "SymbolName"=w857, "WriterMode"=w856, "WriteHandle"=w855, "error constant"=w854, "ADS Write Data"=w810) -> ("Handle"=w850:u32, "WriteHandle"=w849:u32, "Write status?"=w506:bool, "error IO"=w633:errorcluster)  [unwired: 5 in, 1 out]
    n415 = call <userlib>:"Send Writer-Request.vi"("Handle"=w870, "SymbolName"=w869, "WriterMode"=w868, "WriteHandle"=w867, "error constant"=w866, "ADS Write Data"=w811) -> ("Handle"=w862:u32, "WriteHandle"=w861:u32, "Write status?"=w507:bool, "error IO"=w636:errorcluster)  [unwired: 5 in, 1 out]
    n416 = call <userlib>:"Send Writer-Request.vi"("Handle"=w846, "SymbolName"=w845, "WriterMode"=w844, "WriteHandle"=w843, "error constant"=w842, "ADS Write Data"=w809) -> ("Handle"=w838:u32, "WriteHandle"=w837:u32, "Write status?"=w505:bool, "error IO"=w630:errorcluster)  [unwired: 5 in, 1 out]
    n417 = call <userlib>:"Send Writer-Request.vi"("Handle"=w966, "SymbolName"=w965, "WriterMode"=w964, "WriteHandle"=w962, "error constant"=w963, "ADS Write Data"=w819) -> ("Handle"=w961:u32, "WriteHandle"=w960:u32, "Write status?"=w695:bool, "error IO"=w659:errorcluster)  [unwired: 5 in, 1 out]
    n418 = call <userlib>:"Send Writer-Request.vi"("Handle"=w906, "SymbolName"=w905, "WriterMode"=w904, "WriteHandle"=w903, "error constant"=w902, "ADS Write Data"=w814) -> ("Handle"=w898:u32, "WriteHandle"=w897:u32, "Write status?"=w705:bool, "error IO"=w644:errorcluster)  [unwired: 5 in, 1 out]
    n419 = call <userlib>:"Send Writer-Request.vi"("Handle"=w954, "SymbolName"=w953, "WriterMode"=w952, "WriteHandle"=w951, "error constant"=w950, "ADS Write Data"=w818) -> ("Handle"=w946:u32, "WriteHandle"=w945:u32, "Write status?"=w697:bool, "error IO"=w656:errorcluster)  [unwired: 5 in, 1 out]
    n420 = call <userlib>:"Send Writer-Request.vi"("Handle"=w930, "SymbolName"=w929, "WriterMode"=w928, "WriteHandle"=w927, "error constant"=w926, "ADS Write Data"=w816) -> ("Handle"=w922:u32, "WriteHandle"=w921:u32, "Write status?"=w701:bool, "error IO"=w650:errorcluster)  [unwired: 5 in, 1 out]
    n421 = call <userlib>:"Send Writer-Request.vi"("Handle"=w942, "SymbolName"=w941, "WriterMode"=w940, "WriteHandle"=w939, "error constant"=w938, "ADS Write Data"=w817) -> ("Handle"=w934:u32, "WriteHandle"=w933:u32, "Write status?"=w699:bool, "error IO"=w653:errorcluster)  [unwired: 5 in, 1 out]
    n422 = call <userlib>:"Send Writer-Request.vi"("Handle"=w918, "SymbolName"=w917, "WriterMode"=w916, "WriteHandle"=w915, "error constant"=w914, "ADS Write Data"=w815) -> ("Handle"=w910:u32, "WriteHandle"=w909:u32, "Write status?"=w703:bool, "error IO"=w647:errorcluster)  [unwired: 5 in, 1 out]
    n423 = call <userlib>:"Send Writer-Request.vi"("Handle"=w622, "SymbolName"=w621, "WriterMode"=w620, "WriteHandle"=w619, "error constant"=w618, "ADS Write Data"=w614) -> ("Handle"=w613:u32, "WriteHandle"=w612:u32, "Write status?"=w606:bool, "error IO"=w469:errorcluster)  [unwired: 5 in, 1 out]
    n424 = Compound Arithmetic op=AND(w493, w491, w490, w489) -> (w492:bool)
    n425 = And(x=w462, y=w492) -> (x .and. y?=w530:bool)
    n426 = And(x=w452, y=w530) -> (x .and. y?=w604:bool)
    n427 = And(x=w691, y=w604) -> (x .and. y?=w690:bool)
    n428 = And(x=w442, y=w690) -> (x .and. y?=w689:bool)
    n429 = And(x=w688, y=w689) -> (x .and. y?=w687:bool)
    n430 = And(x=w686, y=w687) -> (x .and. y?=w685:bool)
    n431 = And(x=w684, y=w685) -> (x .and. y?=w683:bool)
    n432 = And(x=w682, y=w683) -> (x .and. y?=w681:bool)
    n433 = And(x=w680, y=w681) -> (x .and. y?=w597:bool)
    n434 = And(x=w608, y=w597) -> (x .and. y?=w609:bool)
    n435 = And(x=w679, y=w609) -> (x .and. y?=w678:bool)
    n436 = And(x=w677, y=w678) -> (x .and. y?=w676:bool)
    n437 = And(x=w675, y=w676) -> (x .and. y?=w674:bool)
    n438 = And(x=w673, y=w674) -> (x .and. y?=w672:bool)
    n439 = And(x=w671, y=w672) -> (x .and. y?=w670:bool)
    n440 = And(x=w669, y=w670) -> (x .and. y?=w668:bool)
    n441 = And(x=w667, y=w668) -> (x .and. y?=w666:bool)
    n442 = And(x=w693, y=w666) -> (x .and. y?=→"bHasMached":bool)
    n443 = Compound Arithmetic op=AND(w485, w486, w487, w488) -> (w484:bool)
    n444 = And(x=w460, y=w484) -> (x .and. y?=w531:bool)
    n445 = And(x=w451, y=w531) -> (x .and. y?=w501:bool)
    n446 = Compound Arithmetic op=AND(w509, w508, w507, w506, w505, w441, w504) -> (w503:bool)
    n447 = Not(x=w503) -> (.not. x?=w502:bool)
    n448 = And(x=w502, y=w501) -> (x .and. y?=w500:bool)
    n449 = And(x=w606, y=w500) -> (x .and. y?=w607:bool)
    n450 = And(x=w705, y=w607) -> (x .and. y?=w704:bool)
    n451 = And(x=w703, y=w704) -> (x .and. y?=w702:bool)
    n452 = And(x=w701, y=w702) -> (x .and. y?=w700:bool)
    n453 = And(x=w699, y=w700) -> (x .and. y?=w698:bool)
    n454 = And(x=w697, y=w698) -> (x .and. y?=w696:bool)
    n455 = And(x=w695, y=w696) -> (x .and. y?=w694:bool)
    n456 = And(x=w707, y=w694) -> (x .and. y?=w706:bool)
    n457 = And(x=w708, y=w706) -> (x .and. y?=→"Write Status":bool)
    n458 = feedback #2(TRUE) -> (w553:bool)
    n459 = And(x=w553, y=w556) -> (x .and. y?=w555:bool)
    n460 = feedback #3(TRUE) -> (w563:bool)
    n461 = And(x=w563, y=w566) -> (x .and. y?=w565:bool)
    n462 = feedback #4(TRUE) -> (w567:bool)
    n463 = And(x=w567, y=w570) -> (x .and. y?=w569:bool)
    n464 = feedback #5(TRUE) -> (w559:bool)
    n465 = And(x=w559, y=w558) -> (x .and. y?=w560:bool)
    n466 = case shown="True" w560 {
      tunnel: [w1173 FALSE] -> w550
      tunnel: w551 -> [w1175 _]
      frame False {
        n467 = Or(x=w1175, y=FALSE) -> (x .or. y?=w1173:bool)
      }
      frame True {
        n468 = call "Charge relay error"() -> ()  [unwired: 10 in, 2 out]
      }
    }
    n469 = feedback-in #5(w550) -> ()
    n470 = case shown="True" w555 {
      tunnel: [w1171 FALSE] -> w554
      tunnel: w550 -> [w1169 _]
      frame False {
        n471 = Or(x=w1169, y=FALSE) -> (x .or. y?=w1171:bool)
      }
      frame True {
        n472 = call "PSU HV error"() -> ()  [unwired: 10 in, 2 out]
      }
    }
    n473 = feedback-in #2(w554) -> ()
    n474 = case shown="True" w569 {
      tunnel: [w1182 FALSE] -> w568
      tunnel: w551 -> [w1181 _]
      frame False {
        n475 = Or(x=w1181, y=FALSE) -> (x .or. y?=w1182:bool)
      }
      frame True {
        n476 = call "Softdump error"() -> ()  [unwired: 10 in, 2 out]
      }
    }
    n477 = feedback-in #4(w568) -> ()
    n478 = case shown="True" w565 {
      tunnel: [w1177 FALSE] -> w564
      tunnel: w550 -> [w1178 _]
      frame False {
        n479 = Or(x=w1178, y=FALSE) -> (x .or. y?=w1177:bool)
      }
      frame True {
        n480 = call "Soft Exception"() -> ()  [unwired: 10 in, 2 out]
      }
    }
    n481 = feedback-in #3(w564) -> ()
    n482 = Compound Arithmetic op=OR(w628, w665, w664) -> (w663:bool)
    n483 = Compound Arithmetic op=OR(w663, w662, w661) -> (w660:bool)
    n484 = Compound Arithmetic op=OR(w660, w659, w658) -> (w657:bool)
    n485 = Compound Arithmetic op=OR(w657, w656, w655) -> (w654:bool)
    n486 = Compound Arithmetic op=OR(w654, w653, w652) -> (w651:bool)
    n487 = Compound Arithmetic op=OR(w651, w650, w649) -> (w648:bool)
    n488 = Compound Arithmetic op=OR(w648, w647, w646) -> (w645:bool)
    n489 = Compound Arithmetic op=OR(w645, w644, w643) -> (w605:bool)
    n490 = Compound Arithmetic op=OR(w605, w469, w468) -> (w596:bool)
    n491 = Compound Arithmetic op=OR(w596, w642, w641) -> (w640:bool)
    n492 = Compound Arithmetic op=OR(w640, w639, w638) -> (w637:bool)
    n493 = Compound Arithmetic op=OR(w637, w636, w635) -> (w634:bool)
    n494 = Compound Arithmetic op=OR(w634, w633, w632) -> (w631:bool)
    n495 = Compound Arithmetic op=OR(w631, w630, w629) -> (w443:bool)
    n496 = Compound Arithmetic op=OR(w443, w472, w471) -> (w453:bool)
    n497 = Compound Arithmetic op=OR(w453, "EXIT HMI", w440) -> (w439:bool)
    "Stop Loops" <- w439
    n498 = property on="Stop Loops" class="Bool (strict)"("Val(Sgnl)"=w439) -> ()  [unwired: 2 in, 2 out]
    n499 = node-c288() -> ()  [unwired: 1 in, 1 out]
  }
  n500 = node-c288(w98) -> (w97:errorcluster)
  n501 = call <userlib>:"Release Writer.vi"("Handle"=w268, "WriteHandle"=w267, "error in (no error)"=w266) -> ("error out"=w274:errorcluster)  [unwired: 11 in, 1 out]
  n502 = call <userlib>:"Release Writer.vi"("Handle"=w248, "WriteHandle"=w247, "error in (no error)"=w246) -> ("error out"=w242:errorcluster)  [unwired: 11 in, 1 out]
  n503 = call <userlib>:"Release Writer.vi"("Handle"=w210, "WriteHandle"=w209, "error in (no error)"=w208) -> ("error out"=w204:errorcluster)  [unwired: 11 in, 1 out]
  n504 = call <userlib>:"Release Type.vi"("Handle"=w263, "TypeHandle"=w264, "error in (no error)"=w265) -> ("error out"=w275:errorcluster)  [unwired: 11 in, 1 out]
  n505 = call <userlib>:"Release Type.vi"("Handle"=w245, "TypeHandle"=w244, "error in (no error)"=w243) -> ("error out"=w241:errorcluster)  [unwired: 11 in, 1 out]
  n506 = call <userlib>:"Release Writer.vi"("Handle"=w229, "WriteHandle"=w228, "error in (no error)"=w227) -> ("error out"=w223:errorcluster)  [unwired: 11 in, 1 out]
  n507 = call <userlib>:"Release Type.vi"("Handle"=w207, "TypeHandle"=w206, "error in (no error)"=w205) -> ("error out"=w203:errorcluster)  [unwired: 11 in, 1 out]
  n508 = call <userlib>:"Release Writer.vi"("Handle"=w191, "WriteHandle"=w190, "error in (no error)"=w189) -> ("error out"=w185:errorcluster)  [unwired: 11 in, 1 out]
  n509 = call <userlib>:"Release Type.vi"("Handle"=w226, "TypeHandle"=w225, "error in (no error)"=w224) -> ("error out"=w222:errorcluster)  [unwired: 11 in, 1 out]
  n510 = call <userlib>:"Release Type.vi"("Handle"=w188, "TypeHandle"=w187, "error in (no error)"=w186) -> ("error out"=w184:errorcluster)  [unwired: 11 in, 1 out]
  n511 = call <userlib>:"Release Writer.vi"("Handle"=w417, "WriteHandle"=w416, "error in (no error)"=w427) -> ("error out"=w117:errorcluster)  [unwired: 11 in, 1 out]
  n512 = call <userlib>:"Release Writer.vi"("Handle"=w286, "WriteHandle"=w285, "error in (no error)"=w284) -> ("error out"=w280:errorcluster)  [unwired: 11 in, 1 out]
  n513 = call <userlib>:"Release Writer.vi"("Handle"=w382, "WriteHandle"=w381, "error in (no error)"=w380) -> ("error out"=w388:errorcluster)  [unwired: 11 in, 1 out]
  n514 = call <userlib>:"Release Writer.vi"("Handle"=w362, "WriteHandle"=w361, "error in (no error)"=w360) -> ("error out"=w356:errorcluster)  [unwired: 11 in, 1 out]
  n515 = call <userlib>:"Release Writer.vi"("Handle"=w324, "WriteHandle"=w323, "error in (no error)"=w322) -> ("error out"=w318:errorcluster)  [unwired: 11 in, 1 out]
  n516 = call <userlib>:"Release Type.vi"("Handle"=w283, "TypeHandle"=w282, "error in (no error)"=w281) -> ("error out"=w279:errorcluster)  [unwired: 11 in, 1 out]
  n517 = call <userlib>:"Release Type.vi"("Handle"=w377, "TypeHandle"=w378, "error in (no error)"=w379) -> ("error out"=w389:errorcluster)  [unwired: 11 in, 1 out]
  n518 = call <userlib>:"Release Type.vi"("Handle"=w359, "TypeHandle"=w358, "error in (no error)"=w357) -> ("error out"=w355:errorcluster)  [unwired: 11 in, 1 out]
  n519 = call <userlib>:"Release Writer.vi"("Handle"=w343, "WriteHandle"=w342, "error in (no error)"=w341) -> ("error out"=w337:errorcluster)  [unwired: 11 in, 1 out]
  n520 = call <userlib>:"Release Type.vi"("Handle"=w321, "TypeHandle"=w320, "error in (no error)"=w319) -> ("error out"=w317:errorcluster)  [unwired: 11 in, 1 out]
  n521 = call <userlib>:"Release Writer.vi"("Handle"=w305, "WriteHandle"=w304, "error in (no error)"=w303) -> ("error out"=w299:errorcluster)  [unwired: 11 in, 1 out]
  n522 = call <userlib>:"Release Type.vi"("Handle"=w340, "TypeHandle"=w339, "error in (no error)"=w338) -> ("error out"=w336:errorcluster)  [unwired: 11 in, 1 out]
  n523 = call <userlib>:"Release Type.vi"("Handle"=w302, "TypeHandle"=w301, "error in (no error)"=w300) -> ("error out"=w298:errorcluster)  [unwired: 11 in, 1 out]
  n524 = call <userlib>:"Release Writer.vi"("Handle"=w400, "WriteHandle"=w399, "error in (no error)"=w398) -> ("error out"=w394:errorcluster)  [unwired: 11 in, 1 out]
  n525 = call <userlib>:"Release Writer.vi"("Handle"=w81, "WriteHandle"=w80, "error in (no error)"=w15) -> ("error out"=w95:errorcluster)  [unwired: 11 in, 1 out]
  n526 = call <userlib>:"Release Writer.vi"("Handle"=w17, "WriteHandle"=w153, "error in (no error)"=w20) -> ("Handle"=w9:u32, "error out"=w159:errorcluster)  [unwired: 11 in]
  n527 = call <userlib>:"Release Type.vi"("Handle"=w397, "TypeHandle"=w396, "error in (no error)"=w395) -> ("error out"=w393:errorcluster)  [unwired: 11 in, 1 out]
  n528 = call <userlib>:"Release Type.vi"("Handle"=w79, "TypeHandle"=w78, "error in (no error)"=w14) -> ("error out"=w94:errorcluster)  [unwired: 11 in, 1 out]
  n529 = call <userlib>:"Release Type.vi"("Handle"=w149, "TypeHandle"=w148, "error in (no error)"=w19) -> ("error out"=w158:errorcluster)  [unwired: 11 in, 1 out]
  n530 = call <userlib>:"Release Type.vi"("Handle"=w415, "TypeHandle"=w414, "error in (no error)"=w426) -> ("error out"=w118:errorcluster)  [unwired: 11 in, 1 out]
  n531 = Merge Errors(w274, w275) -> (w106:errorcluster)
  n532 = Merge Errors(w242, w241) -> (w105:errorcluster)
  n533 = Merge Errors(w204, w203) -> (w103:errorcluster)
  n534 = Merge Errors(w223, w222) -> (w104:errorcluster)
  n535 = Merge Errors(w185, w184) -> (w102:errorcluster)
  n536 = Merge Errors(w388, w389) -> (w112:errorcluster)
  n537 = Merge Errors(w280, w279) -> (w107:errorcluster)
  n538 = Merge Errors(w356, w355) -> (w111:errorcluster)
  n539 = Merge Errors(w318, w317) -> (w109:errorcluster)
  n540 = Merge Errors(w337, w336) -> (w110:errorcluster)
  n541 = Merge Errors(w299, w298) -> (w108:errorcluster)
  n542 = Merge Errors(w394, w393) -> (w113:errorcluster)
  n543 = Merge Errors(w95, w94) -> (w93:errorcluster)
  n544 = Merge Errors(w159, w158) -> (w101:errorcluster)
  n545 = Merge Errors(w117, w118) -> (w116:errorcluster)
  n546 = Merge Errors(w49, w48, w47, w46, w38, w21, w2, w1) -> (w44:errorcluster)
  n547 = Merge Errors(w112, w111, w110, w109, w108, w107, w93) -> (w176:errorcluster)
  n548 = Merge Errors(w106, w105, w104, w103, w102, w6, w101, w10, w12, w33, w32, w31, w27) -> (w175:errorcluster)
  n549 = Merge Errors(w128, w129, w130, w131, w132, w74, w73, w69, w70, w71, w72) -> (w119:errorcluster)
  n550 = Merge Errors(w96, w127, w126, w125, w124, w123, w122, w121, w60, w59, w58, w45, w44) -> (w120:errorcluster)
  n551 = Merge Errors(w119, w120) -> (w26:errorcluster)
  n552 = Merge Errors(w97, w116, w113, w176, w175, w26) -> (w114:errorcluster)
  n553 = call <userlib>:"Release.vi"("Handle"=w9, "error in (no error)"=w114) -> ("error out"=→"error out":errorcluster)  [unwired: 13 in]
